vi "SpectrometerSpinCoater_v06.vi"() -> ()   [LabVIEW 2018]
uses:
  <instrlib>/Classes/CCD/Abstract_CCD/Abstract_CCD.lvclass
  TypDef/DeviceQueue_TypeDef.ctl
  TypDef/DeviceQueue_Action.ctl
  TypDef/DataQueue_TypeDef.ctl
  TypDef/DataQueue_Action.ctl
  <vilib>/Utility/error.llb/DialogType.ctl
  <instrlib>/Classes/CCD/Avantes/Avantes.lvclass
  C:/Program Files/National Instruments/LabVIEW 2018/instr.lib/Classes/CCD/Abstract_CCD/Abstract_CCD.lvclass
  <vilib>/Analysis/baseanly.llb/A x Vector.vi
  <vilib>/Instr/_visa.llb/VISA Configure Serial Port (Instr).vi
  <vilib>/Analysis/NI_AALBase.lvlib
panel:
  out "Time.spin":refnum<file>
  out "Meas.spin":refnum<file>
  out "Arduino":bool
  out "NKT":bool
  out "Spectromter":bool
  in  "Abort Button":bool
  in  "Stop Button":bool
  in  "Tab Control":enum32{"Measure", "Settings"}(tab)=enum."Settings"
  in  "Spectra Count":u16
  in  "Measure Spectrum":bool
  out "Action":string
  in  "Preview":bool
  out "XY Graph":T1(graph)
  in  "Frames for Spectrometer":dbl=1.0
  in  "StartSpin_Button":bool
  out "Overall Time":dbl
  in  "Seconds after Spin Stop":dbl[unit]=0.5
  in  "Program Spin Coater\nSpeed (rpm)          Time (s)":dbl[][](array[numeric])
  in  "Record RefSpec":bool
  in  "Record_Darkspec":bool
  in  "Comments":string="Just for testing"
  in  "File Name":string="Temp"
  in  "Save Path":path=path "C:/Users/Timo/Desktop/SpinCoater/Measurement"
  in  "Seconds to Spin Start":dbl[unit]=1.0
  in  "Calculate Frames":bool=TRUE
  in  "Frames":i32
  out "Frame Rate":dbl[unit]
  in  "Integration Time":dbl[unit]=3e-05
  in  "StartMeasurement_Button":bool
  in  "Dividider Get Spectra":u32=1 min=1
  in  "Automatically \nadjust count":bool
  in  "Reset Count\nafter Spin Coating":bool
  in  "Speed":dbl
  in  "Milliseconds":dbl
  in  "Debug":bool
  in  "Port Arduino":refnum<visa-resource-name>="COM6"
  out "Error Arduino":bool caption="Error"
  in  "Init_Arduino":bool=TRUE caption="Init"
  out "Caption_Settings_Arduino":string="Arduino"
  out "Caption_Settings_NKT":string="NKT Laser"
  out "Error_Spectromter":bool caption="Error"
  in  "Init_Spectrometer":bool=TRUE caption="Init"
  out "Caption_Settings_Spectrometer":string="Spectromter"
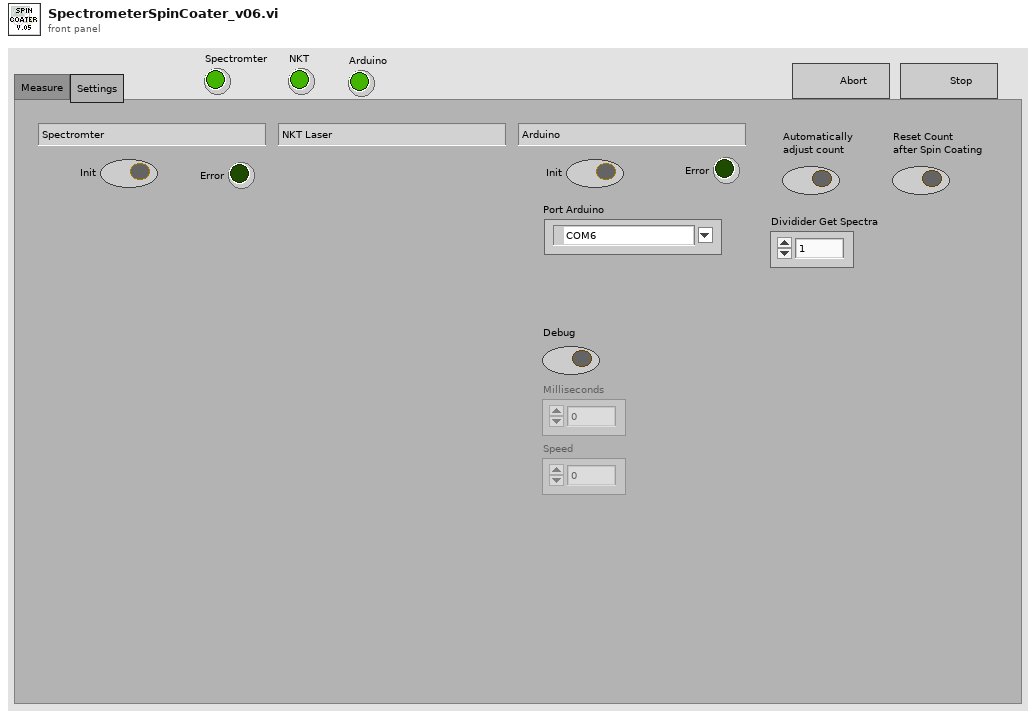
[diagram p1: front panel]
types:
  T1 = cluster{"Wavlength":dbl[unit][], "Image":dbl[]}[]
  T2 = cluster{"Dark":cluster{"Image":dbl[][][], "Frame Size":cluster{"F":i32, "Y":i32, "X":i32}}[], "Ref":cluster{"Image":dbl[][][], "Frame Size":cluster{"F":i32, "Y":i32, "X":i32}}[], "Wavlength":dbl[unit][], "spec":dbl[][]}
  T3 = cluster{"Port Arduino":refnum<visa-resource-name>, "Abstract_CCD.lvclass":refnum<class "Abstract_CCD.lvclass">}
  T4 = typedef "DataQueue_TypeDef.ctl" = cluster{"QueueAction":T5, "Data":cluster{"Image":dbl[][][], "Frame Size":cluster{"F":i32, "Y":i32, "X":i32}}[], "Data_Raw":cluster{"Image":dbl[][][], "Frame Size":cluster{"F":i32, "Y":i32, "X":i32}}[], "Data_Dark":cluster{"Image":dbl[][][], "Frame Size":cluster{"F":i32, "Y":i32, "X":i32}}[], "Data_Ref":cluster{"Image":dbl[][][], "Frame Size":cluster{"F":i32, "Y":i32, "X":i32}}[], "Device Information":string[], "Numeric Control":dbl, "Boolean":bool, "Wavelength":dbl[unit][], "Time":dbl[], "Time Stamp":timestamp, "Numeric Control 2":dbl}
  T5 = typedef "DataQueue_Action.ctl" = enum16{"TimeOut", "Close_Program", "Stop_Measurement", "Measure_InSituSpinCoating", "Measure_Spectrum", "Save_Data", "Set_Ref", "Set_Dark", "Set_Wavelength", "Spectrometer_Measure", "Spectrometer_Preview", "Transfer_Settings"}
  T6 = typedef "DeviceQueue_TypeDef.ctl" = cluster{"QueueAction":T7, "Numeric 1":dbl, "Numeric 2":dbl, "Boolean 1":bool, "Boolean 2":bool, "Spin Program":dbl[][]}
  T7 = typedef "DeviceQueue_Action.ctl" = enum16{"TimeOut", "Close_Program", "Abort", "Spectrometer_Init", "Spectrometer_Close", "Spectrometer_DeviceInformation", "Spectrometer_Measure", "Spectrometer_Preview", "Spectrometer_Abort", "Spectrometer_StartMeasurement", "Spectrometer_GetData", "Spectrometer_StopMeasurement", "Spectrometer_SetIntegrationTime", "Spectrometer_SetFrames", "Spectrometer_SetDarkspec", "Spectrometer_SetReference", "Spectrometer_SetTriggerMode", "Laser_Init", "Laser_Close", "Arduino_Init", "Arduino_Close", "Arduino_LoadProgram", "Arduino_StartProgram", "Arduino_SetSpeed", "Arduino_SetMillis", "Arduino_StopSpin", "Measure_InSitu", "Measure_Spectrum", "Measure_Stop"}
  T8 = enum16{"open", "replace", "create", "open or create", "replace or create", "replace or create with confirmation"}
  T9 = cluster{"Image":dbl[][][], "Frame Size":cluster{"F":i32, "Y":i32, "X":i32}}[]
  T10 = cluster{"Image":dbl[][][], "Frame Size":cluster{"F":i32, "Y":i32, "X":i32}}
  T11 = cluster{"Wavlength":dbl[unit][], "A x Vector":dbl[]}
  T12 = cluster{"Wavlength":dbl[unit][], "A x Vector":dbl[]}[]
  T13 = cluster{u16[][], u16[][], dbl[], "Numeric Control":dbl, "Numeric Control 2":dbl}
  T14 = typedef "DialogType.ctl" = u16
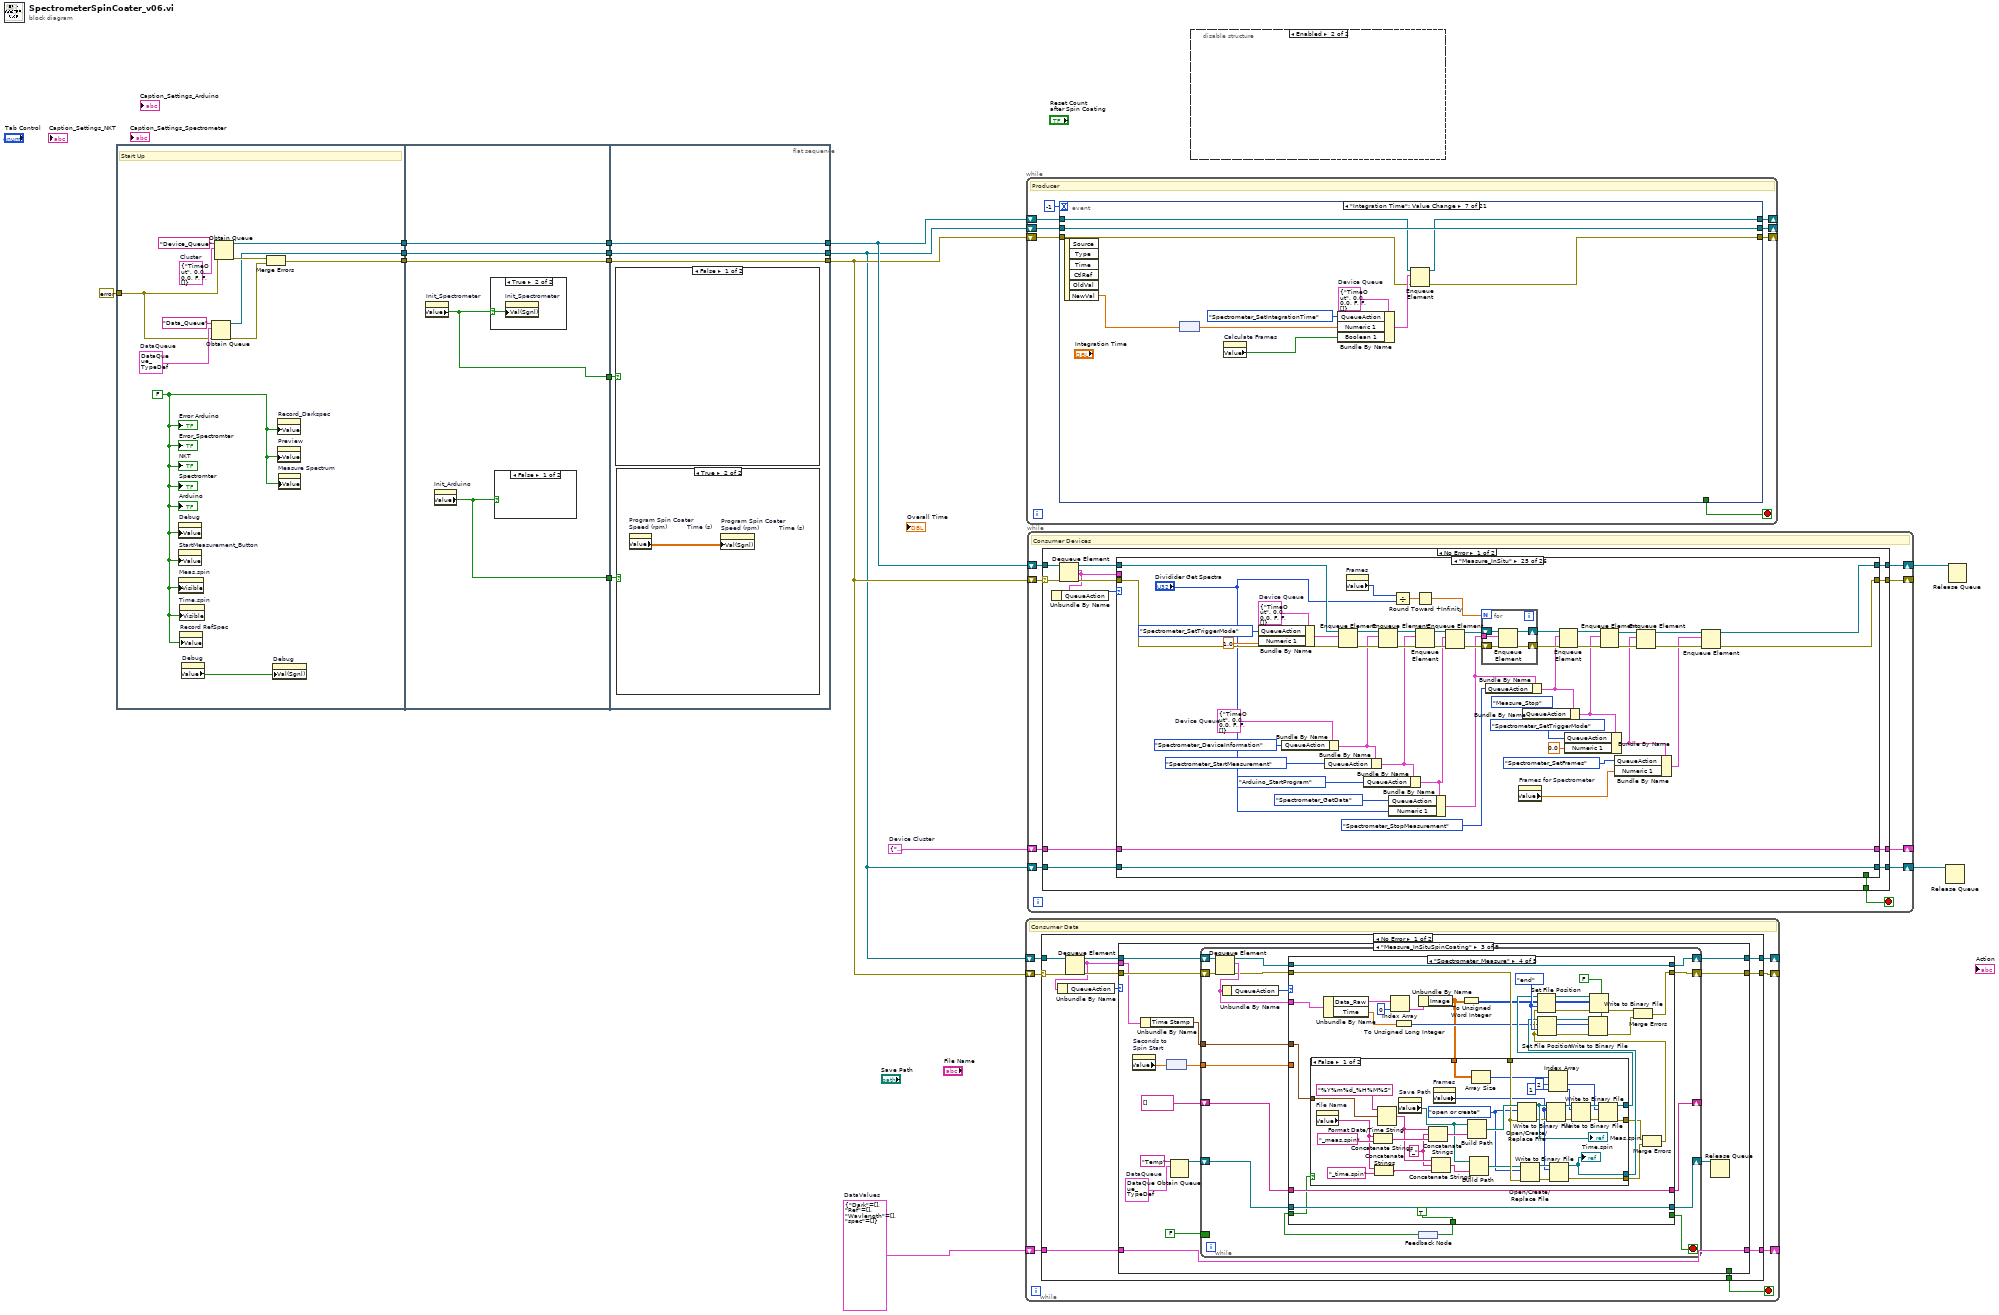
[diagram p0: block diagram]
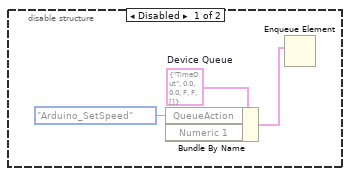
[diagram p2: hidden frame]
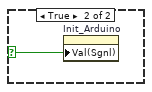
[diagram p3: hidden frame]
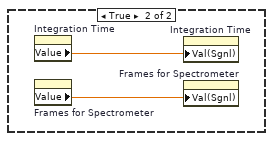
[diagram p6: hidden frame]
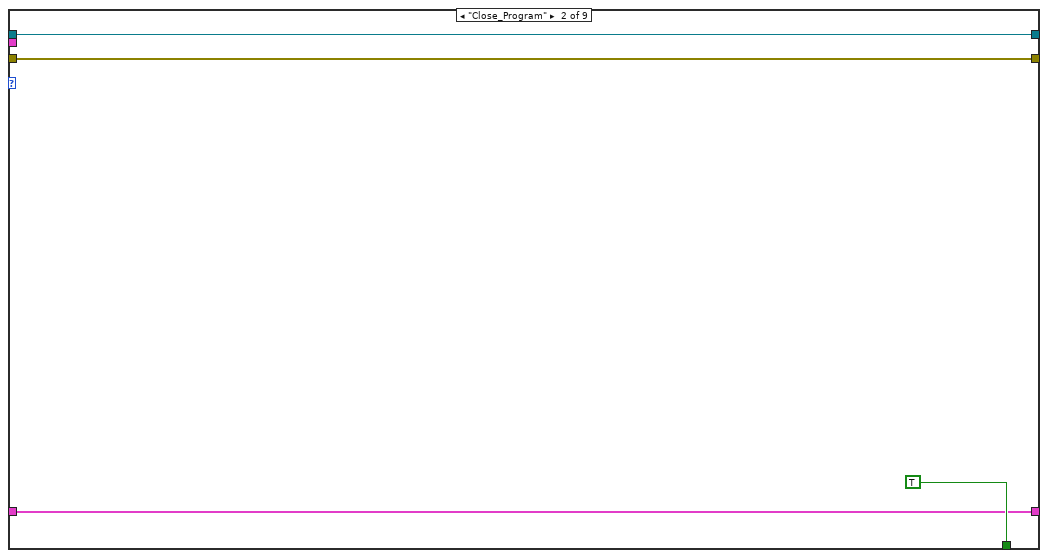
[diagram p8: hidden frame]
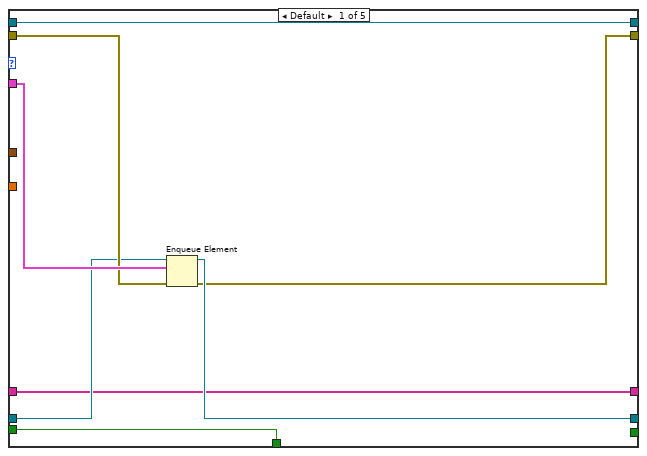
[diagram p9: hidden frame]
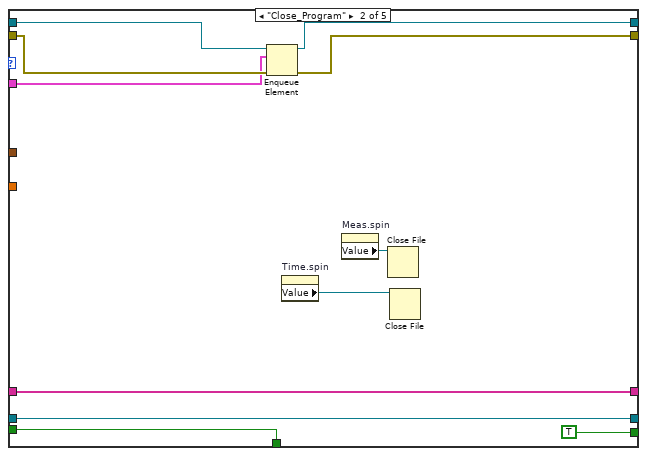
[diagram p10: hidden frame]
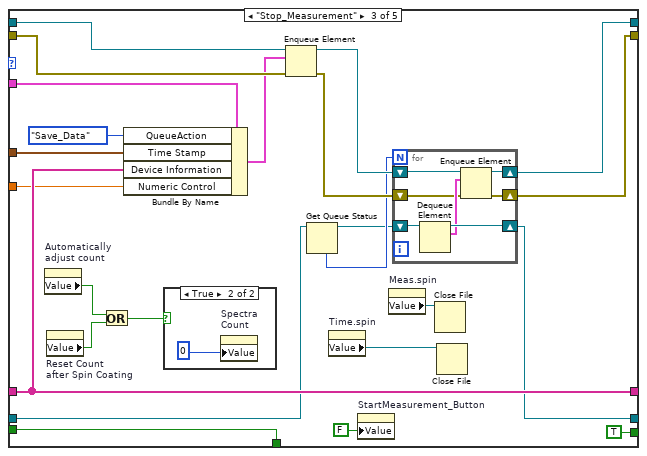
[diagram p11: hidden frame]
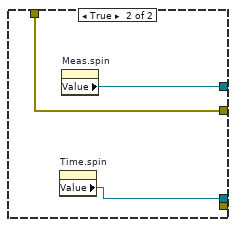
[diagram p13: hidden frame]
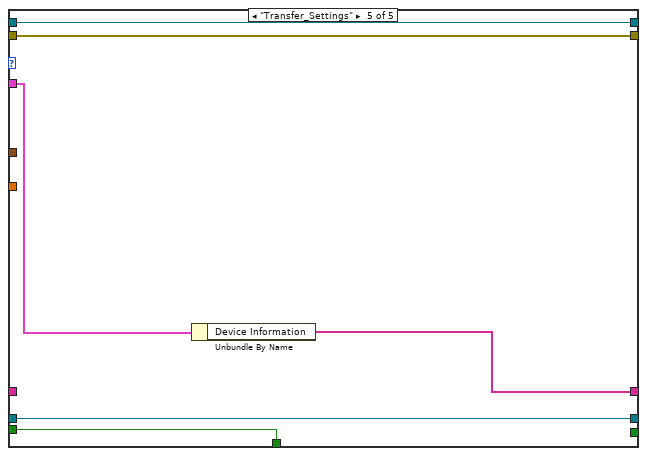
[diagram p14: hidden frame]
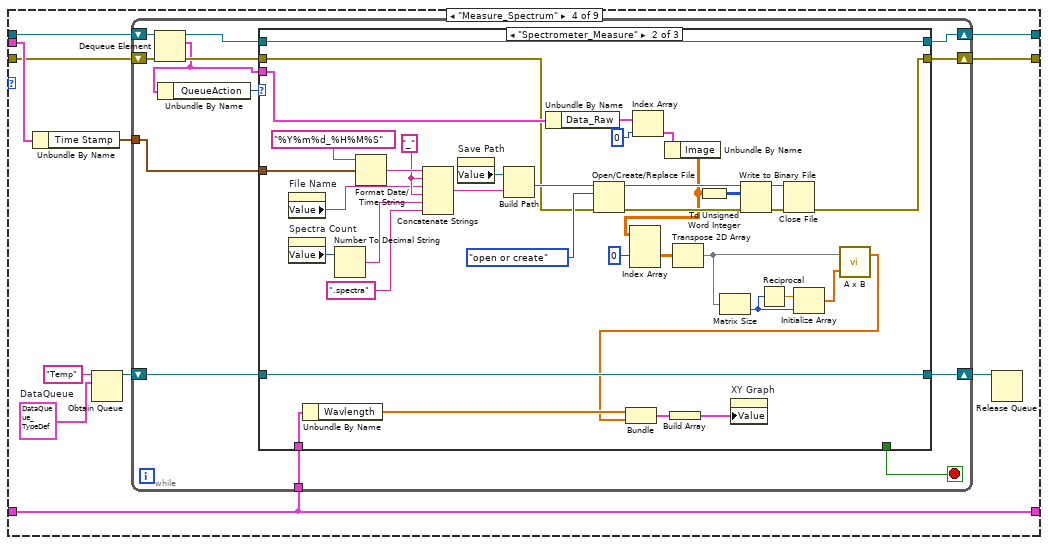
[diagram p15: hidden frame]
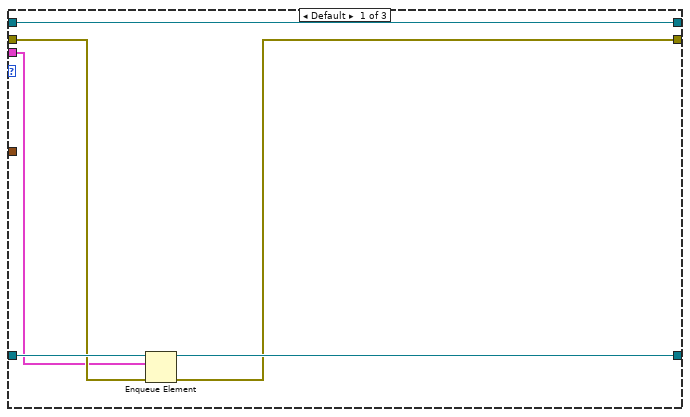
[diagram p16: hidden frame]
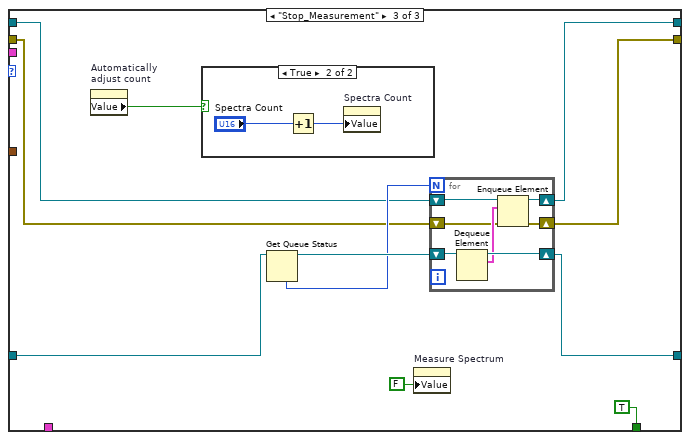
[diagram p17: hidden frame]
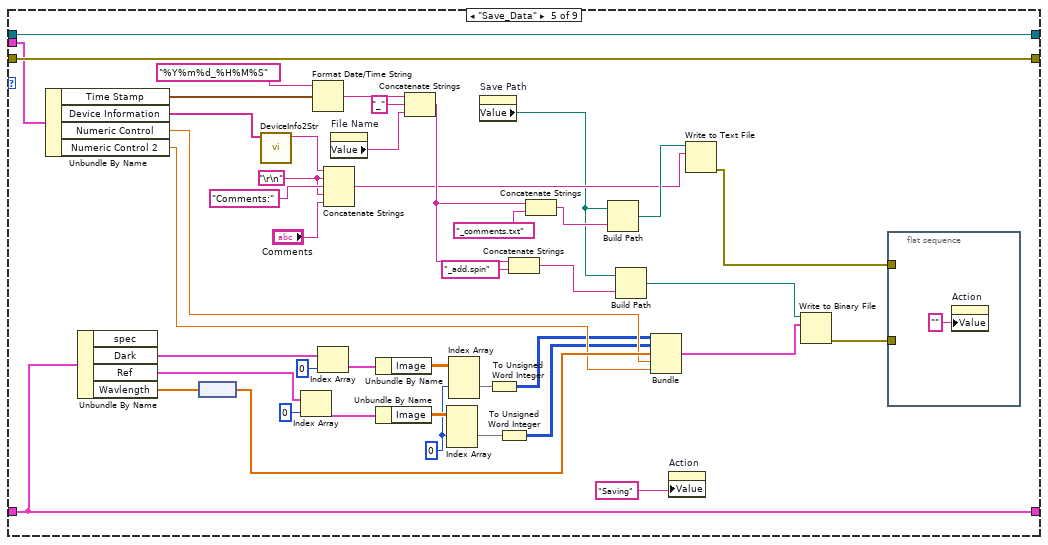
[diagram p19: hidden frame]
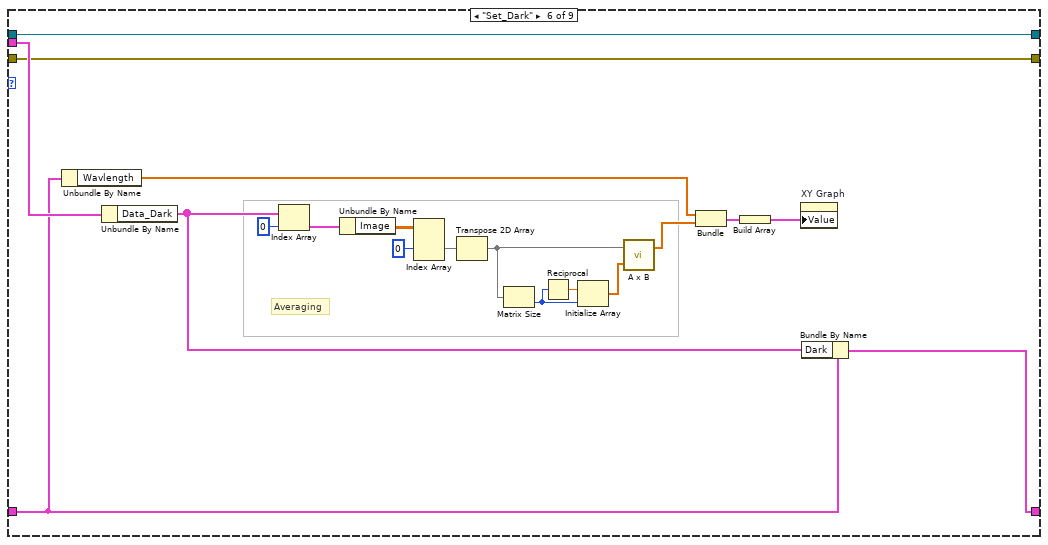
[diagram p20: hidden frame]
diagram:
  w6 = T2 {"Dark"=[], "Ref"=[], "Wavlength"=[], "spec"=[]}  # DataValues
  w11 = T3 {"Port Arduino"="", "Abstract_CCD.lvclass"=refnum}  # Device Cluster
  n1 = flat-sequence {
    tunnel: errorcluster {"status"=FALSE, "code"=0, "source"=""} ("error constant") -> [w23]
    tunnel: [w26] -> w15
    tunnel: [w20] -> w14
    tunnel: [w19] -> w13
    tunnel: w15 -> [w33]
    tunnel: w14 -> [w32]
    tunnel: w13 -> [w31]
    tunnel: [w33] -> w5
    tunnel: [w32] -> w4
    tunnel: [w31] -> w3
    tunnel: [w30] -> w2
    tunnel: [w29] -> w1
    tunnel: [w38] -> w8
    tunnel: [w39] -> w7
    tunnel: [w40] -> w12
    tunnel: w5 -> [w40]
    tunnel: w4 -> [w39]
    tunnel: w3 -> [w38]
    tunnel: w2 -> [w37]
    tunnel: w1 -> [w36]
    frame #0 {
      w24 = T4 {"QueueAction"=enum."TimeOut", "Data"=[], "Data_Raw"=[], "Data_Dark"=[], "Data_Ref"=[], "Device Information"=[], "Numeric Control"=0.0, "Boolean"=FALSE, "Wavelength"=[], "Time"=[], "Time Stamp"=timestamp(0 s since 1904-01-01), "Numeric Control 2"=0.0}  # DataQueue
      w27 = T6 {"QueueAction"=enum."TimeOut", "Numeric 1"=0.0, "Numeric 2"=0.0, "Boolean 1"=FALSE, "Boolean 2"=FALSE, "Spin Program"=[]}  # Cluster
      w18 = FALSE ("Error Arduino")
      # "Start Up"
      n2 = property on="Debug" class="Bool (strict)"("Value"=w18) -> ()  [unwired: 2 in, 2 out]
      n3 = property on="StartMeasurement_Button" class="Bool (strict)"("Value"=w18) -> ()  [unwired: 2 in, 2 out]
      n4 = property on="Meas.spin" class="Ref (strict)"("Visible"=w18) -> ()  [unwired: 2 in, 2 out]
      n5 = property on="Time.spin" class="Ref (strict)"("Visible"=w18) -> ()  [unwired: 2 in, 2 out]
      n6 = property on="Record RefSpec" class="Bool (strict)"("Value"=w18) -> ()  [unwired: 2 in, 2 out]
      n7 = property on="Debug" class="Bool (strict)"() -> ("Value"=w17:bool)  [unwired: 2 in, 2 out]
      n8 = Obtain Queue(name (unnamed)="Data_Queue", element data type=w24, error in (no error)=w23) -> (queue out=w20:refnum<queue>, error out=w21:errorcluster)  [unwired: 2 in, 1 out]
      n9 = Obtain Queue(name (unnamed)="Device_Queue", element data type=w27, error in (no error)=w23) -> (queue out=w26:refnum<queue>, error out=w22:errorcluster)  [unwired: 2 in, 1 out]
      n10 = Merge Errors(w22, w21) -> (w19:errorcluster)
      n11 = property on="Debug" class="Bool (strict)"("Val(Sgnl)"=w17) -> ()  [unwired: 2 in, 2 out]
      n12 = property on="Record_Darkspec" class="Bool (strict)"("Value"=w18) -> ()  [unwired: 2 in, 2 out]
      n13 = property on="Preview" class="Bool (strict)"("Value"=w18) -> ()  [unwired: 2 in, 2 out]
      n14 = property on="Measure Spectrum" class="Bool (strict)"("Value"=w18) -> ()  [unwired: 2 in, 2 out]
      "Error_Spectromter" <- w18
      "Error Arduino" <- w18
      "Spectromter" <- w18
      "NKT" <- w18
      "Arduino" <- w18
    }
    frame #1 {
      n15 = property on="Init_Spectrometer" class="Bool (strict)"() -> ("Value"=w30:bool)  [unwired: 2 in, 2 out]
      n16 = property on="Init_Arduino" class="Bool (strict)"() -> ("Value"=w29:bool)  [unwired: 2 in, 2 out]
      n17 = case shown="True" w30 {
        selector: w30 -> [_ w35]
        frame False {
        }
        frame True {
          n18 = property on="Init_Spectrometer" class="Bool (strict)"("Val(Sgnl)"=w35) -> ()  [unwired: 2 in, 2 out]
        }
      }
      n19 = case shown="False" w29 {
        selector: w29 -> [_ w34]
        frame False {
        }
        frame True {
          n20 = property on="Init_Arduino" class="Bool (strict)"("Val(Sgnl)"=w34) -> ()  [unwired: 2 in, 2 out]
        }
      }
    }
    frame #2 {
      n21 = case shown="False" w37 {
        frame False {
        }
        frame True {
          n22 = property on="Integration Time" class="DigNum (strict)"() -> ("Value"=w42:dbl[unit])  [unwired: 2 in, 2 out]
          n23 = property on="Frames for Spectrometer" class="DigNum (strict)"() -> ("Value"=w43:dbl)  [unwired: 2 in, 2 out]
          n24 = property on="Integration Time" class="DigNum (strict)"("Val(Sgnl)"=w42) -> ()  [unwired: 2 in, 2 out]
          n25 = property on="Frames for Spectrometer" class="DigNum (strict)"("Val(Sgnl)"=w43) -> ()  [unwired: 2 in, 2 out]
        }
      }
      n26 = case shown="True" w36 {
        frame False {
        }
        frame True {
          n27 = property on="Program Spin Coater\nSpeed (rpm)          Time (s)" class="Arr (strict)"() -> ("Value"=w41:dbl[][])  [unwired: 2 in, 2 out]
          n28 = property on="Program Spin Coater\nSpeed (rpm)          Time (s)" class="Arr (strict)"("Val(Sgnl)"=w41) -> ()  [unwired: 2 in, 2 out]
        }
      }
    }
  }
  n29 = while {
    shift-right: [w44] -> _
    shift-left: w8 -> [w50]
    shift-right: [w45] -> _
    shift-left: w7 -> [w49]
    shift-right: [w46] -> _
    shift-left: w6 -> [w48]
    stop <- w47 stop-if-true
    # "Consumer Data"
    n30 = case shown="No Error" w50 {
      selector: w50 -> [w61 w416]
      tunnel: w49 -> [w60 w417]
      tunnel: w48 -> [w58 w414]
      tunnel: [w57 _] -> w47
      tunnel: [w56 w414] -> w46
      tunnel: [w55 w417] -> w45
      tunnel: [w53 w415] -> w44
      frame No Error {
        n31 = Dequeue Element(queue=w60, error in (no error)=w61) -> (queue out=w54:refnum<queue>, element=w51:T4, error out=w52:errorcluster)  [unwired: 1 in, 1 out]
        n32 = Unbundle By Name(w51) -> ("QueueAction"=w59:T5)
        n33 = case shown="\"Measure_InSituSpinCoating\"" w59 {
          tunnel: w58 -> [w62 w67 w73 w225 w325 w368 w377 w399 w410]
          tunnel: [_ TRUE _ _ _ _ _ _ _] -> w57
          tunnel: [w62 w67 w73 w225 w325 w372 w391 w398 w410] -> w56
          tunnel: [w64 w66 w83 w231 w355 w373 w392 w395 w413] -> w55
          tunnel: w54 -> [w64 w66 w81 w233 w355 w373 w392 w395 w413]
          tunnel: [w63 w65 w82 w230 w354 w374 w393 w396 w412] -> w53
          tunnel: w52 -> [w63 w65 w80 w234 w354 w374 w393 w396 w412]
          tunnel: w51 -> [_ _ w75 w235 w341 w375 w394 w397 w411]
          frame "TimeOut", Default {
          }
          frame "Close_Program" {
          }
          frame "Measure_InSituSpinCoating" {
            w78 = T4 {"QueueAction"=enum."TimeOut", "Data"=[], "Data_Raw"=[], "Data_Dark"=[], "Data_Ref"=[], "Device Information"=[], "Numeric Control"=0.0, "Boolean"=FALSE, "Wavelength"=[], "Time"=[], "Time Stamp"=timestamp(0 s since 1904-01-01), "Numeric Control 2"=0.0}  # DataQueue
            n34 = property on="Seconds to\nSpin Start" class="DigNum (strict)"() -> ("Value"=w70:dbl[unit])  [unwired: 2 in, 2 out]
            n35 = Unbundle By Name(w75) -> ("Time Stamp"=w74:timestamp)
            n36 = node(w70) -> (w69:dbl)
            n37 = Obtain Queue(name (unnamed)="Temp", element data type=w78) -> (queue out=w77:refnum<queue>)  [unwired: 3 in, 2 out]
            n38 = while {
              shift-right: [w91] -> w83
              shift-left: w81 -> [w100]
              shift-right: [w92] -> w82
              shift-left: w80 -> [w99]
              shift-right: [w93] -> w76
              shift-left: w77 -> [w94]
              tunnel: w74 -> [w87]
              shift-right: [w88] -> _
              shift-left: string[] [] ("Device Information") -> [w89]
              border: FALSE -> [_]
              tunnel: w69 -> [w84]
              stop <- w90 stop-if-true
              n39 = Dequeue Element(queue=w100, error in (no error)=w99) -> (queue out=w95:refnum<queue>, element=w97:T4, error out=w96:errorcluster)  [unwired: 1 in, 1 out]
              n40 = Unbundle By Name(w97) -> ("QueueAction"=w98:T5)
              n41 = feedback #1() -> (w86:bool)
              n42 = case shown="\"Spectrometer_Measure\"" w98 {
                tunnel: w97 -> [w108 w117 w142 w179 w223]
                tunnel: w96 -> [w107 w118 w139 w170 w220]
                tunnel: w95 -> [w103 w119 w138 w178 w221]
                tunnel: w94 -> [w106 w114 w133 w167 w224]
                tunnel: [w105 w114 w130 w167 w224] -> w93
                tunnel: [w104 w115 w129 w168 w220] -> w92
                tunnel: [w103 w116 w128 w178 w221] -> w91
                tunnel: [_ TRUE TRUE _ _] -> w90
                tunnel: w89 -> [w102 w112 w140 w165 _]
                tunnel: [w102 w112 w140 w165 w222] -> w88
                tunnel: w87 -> [_ _ w141 w180 _]
                tunnel: w86 -> [w101 w111 w127 w163 w219]
                tunnel: [w101 w111 w127 TRUE w219] -> w85
                tunnel: w84 -> [_ _ w124 _ _]
                frame Default {
                  n43 = Enqueue Element(queue=w106, element=w108, error in (no error)=w107) -> (queue out=w105:refnum<queue>, error out=w104:errorcluster)  [unwired: 1 in, 1 out]
                }
                frame "Close_Program" {
                  n44 = Enqueue Element(queue=w119, element=w117, error in (no error)=w118) -> (queue out=w116:refnum<queue>, error out=w115:errorcluster)  [unwired: 1 in, 1 out]
                  n45 = property on="Time.spin" class="Ref (strict)"() -> ("Value"=w109:refnum<file>)  [unwired: 2 in, 2 out]
                  n46 = property on="Meas.spin" class="Ref (strict)"() -> ("Value"=w110:refnum<file>)  [unwired: 2 in, 2 out]
                  n47 = Close File(refnum=w110) -> ()  [unwired: 1 in, 2 out]
                  n48 = Close File(refnum=w109) -> ()  [unwired: 1 in, 2 out]
                }
                frame "Stop_Measurement" {
                  n49 = property on="Automatically \nadjust count" class="Bool (strict)"() -> ("Value"=w121:bool)  [unwired: 2 in, 2 out]
                  n50 = property on="Reset Count\nafter Spin Coating" class="Bool (strict)"() -> ("Value"=w122:bool)  [unwired: 2 in, 2 out]
                  n51 = Or(x=w121, y=w122) -> (x .or. y?=w120:bool)
                  n52 = Bundle By Name(cluster=w142, "QueueAction"=DataQueue_Action."Save_Data", "Time Stamp"=w141, "Device Information"=w140, "Numeric Control"=w124) -> (w137:T4)
                  n53 = case shown="True" w120 {
                    frame False {
                    }
                    frame True {
                      n54 = property on="Spectra \nCount" class="DigNum (strict)"("Value"=u16 0 ("Spectra Count")) -> ()  [unwired: 2 in, 2 out]
                    }
                  }
                  n55 = Enqueue Element(queue=w138, element=w137, error in (no error)=w139) -> (queue out=w135:refnum<queue>, error out=w134:errorcluster)  [unwired: 1 in, 1 out]
                  n56 = Get Queue Status(queue=w133) -> (queue out=w131:refnum<queue>, # elements in queue=w132:i32)  [unwired: 2 in, 6 out]
                  n57 = property on="Time.spin" class="Ref (strict)"() -> ("Value"=w125:refnum<file>)  [unwired: 2 in, 2 out]
                  n58 = property on="StartMeasurement_Button" class="Bool (strict)"("Value"=FALSE ("StartMeasurement_Button")) -> ()  [unwired: 2 in, 2 out]
                  n59 = property on="Meas.spin" class="Ref (strict)"() -> ("Value"=w126:refnum<file>)  [unwired: 2 in, 2 out]
                  n60 = for {
                    N: w132 -> [_]
                    shift-right: [w150] -> w130
                    shift-left: w131 -> [w151]
                    shift-right: [w147] -> w128
                    shift-left: w135 -> [w148]
                    shift-right: [w145] -> w129
                    shift-left: w134 -> [w146]
                    n61 = Dequeue Element(queue=w151) -> (queue out=w150:refnum<queue>, element=w149:T4)  [unwired: 2 in, 2 out]
                    n62 = Enqueue Element(queue=w148, element=w149, error in (no error)=w146) -> (queue out=w147:refnum<queue>, error out=w145:errorcluster)  [unwired: 1 in, 1 out]
                  }
                  n63 = Close File(refnum=w126) -> ()  [unwired: 1 in, 2 out]
                  n64 = Close File(refnum=w125) -> ()  [unwired: 1 in, 2 out]
                }
                frame "Spectrometer_Measure" {
                  w153 = FALSE ("prepend array or string size? (T)")
                  w166 = enum16{"start", "end", "current"}."end" ("from (0:start)")
                  n65 = Unbundle By Name(w179) -> ("Data_Raw"=w175:T9, "Time"=w169:dbl[])
                  n66 = Index Array(array=w175, index=0) -> (element=w174:T10)
                  n67 = To Unsigned Long Integer(number=w169) -> (unsigned 32bit integer=w155:u32[])
                  n68 = Unbundle By Name(w174) -> ("Image"=w152:dbl[][][])
                  n69 = case shown="False" w163 {
                    tunnel: w180 -> [w212 _]
                    tunnel: w170 -> [w207 w218]
                    tunnel: [w193 w218] -> w157
                    tunnel: [w181 _] -> w158
                    tunnel: [w192 w217] -> w160
                    tunnel: [w182 w216] -> w159
                    tunnel: w152 -> [w190 _]
                    frame False {
                      w202 = T8."open or create" ("operation (0:open)")
                      w201 = "_" ("string")
                      n70 = property on="File Name" class="Str"() -> ("Value"=w210:string)  [unwired: 2 in, 2 out]
                      n71 = Concatenate Strings(w210, "_meas.spin" ("string")) -> (w213:string)
                      n72 = Concatenate Strings(w210, "_time.spin" ("string")) -> (w205:string)
                      n73 = Format Date/Time String(time format string (%c)="%Y%m%d_%H%M%S", seconds (now)=w212) -> (date/time string=w206:string)  [unwired: 1 in]
                      n74 = property on="Save Path" class="Path"() -> ("Value"=w184:path)  [unwired: 2 in, 2 out]
                      n75 = Concatenate Strings(w206, w201, w213) -> (w211:string)
                      n76 = Concatenate Strings(w206, w201, w205) -> (w204:string)
                      n77 = property on="Frames" class="DigNum (strict)"() -> ("Value"=w183:i32)  [unwired: 2 in, 2 out]
                      n78 = Build Path(base path=w184, name or relative path=w211) -> (appended path=w208:path)
                      n79 = Build Path(base path=w184, name or relative path=w204) -> (appended path=w203:path)
                      n80 = Array Size(array=w190) -> (size(s)=w189:i32[])
                      n81 = Open/Create/Replace File(file path (use dialog)=w208, error in=w207, operation (0:open)=w202) -> (refnum out=w200:refnum<file>, error out=w199:errorcluster)  [unwired: 3 in, 1 out]
                      "Meas.spin" <- w200
                      n82 = Open/Create/Replace File(file path (use dialog)=w203, error in=w207, operation (0:open)=w202) -> (refnum out=w198:refnum<file>, error out=w197:errorcluster)  [unwired: 3 in, 1 out]
                      n83 = Write to Binary File(file (use dialog)=w200, data=w183, error in=w199) -> (refnum out=w196:refnum<file>, error out=w195:errorcluster)  [unwired: 3 in, 1 out]
                      n84 = Index Array(array=w189, index #1=2 ("index"), index #2=1 ("index")) -> (element #1=w185:i32, element #2=w186:i32)
                      n85 = Write to Binary File(file (use dialog)=w198, data=w183, error in=w197) -> (refnum out=w182:refnum<file>, error out=w181:errorcluster)  [unwired: 3 in, 1 out]
                      "Time.spin" <- w182
                      n86 = Write to Binary File(file (use dialog)=w196, data=w186, error in=w195) -> (refnum out=w191:refnum<file>, error out=w194:errorcluster)  [unwired: 3 in, 1 out]
                      n87 = Write to Binary File(file (use dialog)=w191, data=w185, error in=w194) -> (refnum out=w192:refnum<file>, error out=w193:errorcluster)  [unwired: 3 in, 1 out]
                    }
                    frame True {
                      n88 = property on="Time.spin" class="Ref (strict)"() -> ("Value"=w216:refnum<file>)  [unwired: 2 in, 2 out]
                      n89 = property on="Meas.spin" class="Ref (strict)"() -> ("Value"=w217:refnum<file>)  [unwired: 2 in, 2 out]
                    }
                  }
                  n90 = To Unsigned Word Integer(number=w152) -> (unsigned 16bit integer=w154:u16[][][])
                  n91 = Merge Errors(w157, w158) -> (w156:errorcluster)
                  n92 = Set File Position(refnum=w160, from (0:start)=w166, error in=w156) -> (refnum out=w172:refnum<file>, error out=w171:errorcluster)  [unwired: 1 in]
                  n93 = Set File Position(refnum=w159, from (0:start)=w166, error in=w156) -> (refnum out=w177:refnum<file>, error out=w176:errorcluster)  [unwired: 1 in]
                  n94 = Write to Binary File(file (use dialog)=w177, data=w155, error in=w176, 5:w153) -> (error out=w161:errorcluster)  [unwired: 2 in, 2 out]
                  n95 = Write to Binary File(file (use dialog)=w172, data=w154, error in=w171, 5:w153) -> (error out=w162:errorcluster)  [unwired: 2 in, 2 out]
                  n96 = Merge Errors(w162, w161) -> (w168:errorcluster)
                }
                frame "Transfer_Settings" {
                  n97 = Unbundle By Name(w223) -> ("Device Information"=w222:string[])
                }
              }
              n98 = feedback-in #1(w85) -> ()
            }
            n99 = Release Queue(queue=w76) -> ()  [unwired: 2 in, 3 out]
          }
          frame "Measure_Spectrum" {
            w228 = T4 {"QueueAction"=enum."TimeOut", "Data"=[], "Data_Raw"=[], "Data_Dark"=[], "Data_Ref"=[], "Device Information"=[], "Numeric Control"=0.0, "Boolean"=FALSE, "Wavelength"=[], "Time"=[], "Time Stamp"=timestamp(0 s since 1904-01-01), "Numeric Control 2"=0.0}  # DataQueue
            n100 = Unbundle By Name(w235) -> ("Time Stamp"=w232:timestamp)
            n101 = Obtain Queue(name (unnamed)="Temp", element data type=w228) -> (queue out=w227:refnum<queue>)  [unwired: 3 in, 2 out]
            n102 = while {
              shift-right: [w239] -> w231
              shift-left: w233 -> [w247]
              shift-right: [w240] -> w230
              shift-left: w234 -> [w248]
              tunnel: w232 -> [w237]
              shift-right: [w241] -> w226
              shift-left: w227 -> [w243]
              tunnel: w225 -> [w236]
              stop <- w238 stop-if-true
              n103 = Dequeue Element(queue=w247, error in (no error)=w248) -> (queue out=w245:refnum<queue>, element=w242:T4, error out=w244:errorcluster)  [unwired: 1 in, 1 out]
              n104 = Unbundle By Name(w242) -> ("QueueAction"=w246:T5)
              n105 = case shown="\"Spectrometer_Measure\"" w246 {
                tunnel: w245 -> [w249 w267 w298]
                tunnel: w244 -> [w252 w277 w297]
                tunnel: w243 -> [w254 w289 w300]
                tunnel: w242 -> [w250 w291 _]
                tunnel: [w253 w289 w296] -> w241
                tunnel: [w251 w268 w294] -> w240
                tunnel: [w249 w267 w295] -> w239
                tunnel: [_ _ TRUE] -> w238
                tunnel: w237 -> [_ w288 _]
                tunnel: w236 -> [_ w259 _]
                frame Default {
                  n106 = Enqueue Element(queue=w254, element=w250, error in (no error)=w252) -> (queue out=w253:refnum<queue>, error out=w251:errorcluster)  [unwired: 1 in, 1 out]
                }
                frame "Spectrometer_Measure" {
                  w285 = "_"
                  n107 = property on="File Name" class="Str"() -> ("Value"=w284:string)  [unwired: 2 in, 2 out]
                  n108 = property on="Spectra Count" class="DigNum (strict)"() -> ("Value"=w290:u16)  [unwired: 2 in, 2 out]
                  n109 = Unbundle By Name(w259) -> ("Wavlength"=w256:dbl[unit][])
                  n110 = Number To Decimal String(number=w290) -> (decimal integer string=w283:string)  [unwired: 1 in]
                  n111 = Format Date/Time String(time format string (%c)="%Y%m%d_%H%M%S", seconds (now)=w288) -> (date/time string=w286:string)  [unwired: 1 in]
                  n112 = Concatenate Strings(w286, w285, w284, w285, w283, ".spectra" ("string")) -> (w281:string)
                  n113 = property on="Save Path" class="Path"() -> ("Value"=w280:path)  [unwired: 2 in, 2 out]
                  n114 = Build Path(base path=w280, name or relative path=w281) -> (appended path=w279:path)
                  n115 = Unbundle By Name(w291) -> ("Data_Raw"=w274:T9)
                  n116 = Open/Create/Replace File(file path (use dialog)=w279, error in=w277, operation (0:open)=T8."open or create") -> (refnum out=w276:refnum<file>, error out=w275:errorcluster)  [unwired: 3 in, 1 out]
                  n117 = Index Array(array=w274, index=0) -> (element=w272:T10)
                  n118 = Unbundle By Name(w272) -> ("Image"=w260:dbl[][][])
                  n119 = Index Array(array=w260, index (dim 1)=0 ("disabled index (row)")) -> (element=w266:dbl[][])  [unwired: 2 in]
                  n120 = Transpose 2D Array(2D array=w266) -> (transposed array=w263:dbl[][])
                  n121 = To Unsigned Word Integer(number=w260) -> (unsigned 16bit integer=w271:u16[][][])
                  n122 = Matrix Size(0:w263) -> (2:w264:i32)  [unwired: 1 out]
                  n123 = Write to Binary File(file (use dialog)=w276, data=w271, error in=w275) -> (refnum out=w269:refnum<file>, error out=w270:errorcluster)  [unwired: 3 in, 1 out]
                  n124 = Reciprocal(x=w264) -> (1/x=w265:dbl)
                  n125 = Close File(refnum=w269, error in=w270) -> (error out=w268:errorcluster)  [unwired: 1 out]
                  n126 = Initialize Array(w265, w264) -> (w262:dbl[])
                  n127 = call-poly <vilib>:"A x B.vi"("Vector"=w262, "A"=w263) -> ("A x Vector"=w255:dbl[])  [unwired: 1 out]
                  n128 = Bundle("Wavlength"=w256, "A x Vector"=w255) -> (w258:T11)  [unwired: 1 in]
                  n129 = Build Array(w258) -> (w257:T12)
                  n130 = property on="XY Graph" class="XYGraph (strict)"("Value"=w257) -> ()  [unwired: 2 in, 2 out]
                }
                frame "Stop_Measurement" {
                  n131 = property on="Automatically \nadjust count" class="Bool (strict)"() -> ("Value"=w292:bool)  [unwired: 2 in, 2 out]
                  n132 = case shown="True" w292 {
                    frame False {
                    }
                    frame True {
                      n133 = Increment(x="Spectra Count") -> (x+1=w303:u16)
                      n134 = property on="Spectra Count" class="DigNum (strict)"("Value"=w303) -> ()  [unwired: 2 in, 2 out]
                    }
                  }
                  n135 = Get Queue Status(queue=w300) -> (queue out=w301:refnum<queue>, # elements in queue=w299:i32)  [unwired: 2 in, 6 out]
                  n136 = property on="Measure Spectrum" class="Bool (strict)"("Value"=FALSE ("Measure Spectrum")) -> ()  [unwired: 2 in, 2 out]
                  n137 = for {
                    N: w299 -> [_]
                    shift-right: [w310] -> w296
                    shift-left: w301 -> [w311]
                    shift-right: [w307] -> w295
                    shift-left: w298 -> [w308]
                    shift-right: [w305] -> w294
                    shift-left: w297 -> [w306]
                    n138 = Dequeue Element(queue=w311) -> (queue out=w310:refnum<queue>, element=w309:T4)  [unwired: 2 in, 2 out]
                    n139 = Enqueue Element(queue=w308, element=w309, error in (no error)=w306) -> (queue out=w307:refnum<queue>, error out=w305:errorcluster)  [unwired: 1 in, 1 out]
                  }
                }
              }
            }
            n140 = Release Queue(queue=w226) -> ()  [unwired: 2 in, 3 out]
          }
          frame "Save_Data" {
            w327 = "\r\n"
            w314 = 0 ("index (page)")
            n141 = Unbundle By Name(w341) -> ("Time Stamp"=w339:timestamp, "Device Information"=w330:string[], "Numeric Control"=w324:dbl, "Numeric Control 2"=w323:dbl)
            n142 = Unbundle By Name(w325) -> ("Dark"=w351:T9, "Ref"=w349:T9, "Wavlength"=w353:dbl[unit][])  [unwired: 1 out]
            n143 = node(w353) -> (w342:dbl[])
            n144 = call "DeviceInfo2Str.vi"("Device Information"=w330) -> ("String"=w329:string)  [unwired: 10 in]
            n145 = Index Array(array=w349, index=0) -> (element=w347:T10)
            n146 = Format Date/Time String(time format string (%c)="%Y%m%d_%H%M%S", seconds (now)=w339) -> (date/time string=w338:string)  [unwired: 1 in]
            n147 = Index Array(array=w351, index=0) -> (element=w348:T10)
            n148 = Concatenate Strings(w329, w327, "Comments:" ("string"), w327, "Comments") -> (w322:string)
            n149 = property on="File Name" class="Str"() -> ("Value"=w320:string)  [unwired: 2 in, 2 out]
            n150 = Unbundle By Name(w348) -> ("Image"=w346:dbl[][][])
            n151 = Unbundle By Name(w347) -> ("Image"=w345:dbl[][][])
            n152 = Concatenate Strings(w338, "_" ("string"), w320) -> (w336:string)
            n153 = Index Array(array=w345, index (dim 1)=w314) -> (element=w343:dbl[][])  [unwired: 2 in]
            n154 = Index Array(array=w346, index (dim 1)=w314) -> (element=w344:dbl[][])  [unwired: 2 in]
            n155 = property on="Save Path" class="Path"() -> ("Value"=w319:path)  [unwired: 2 in, 2 out]
            n156 = To Unsigned Word Integer(number=w344) -> (unsigned 16bit integer=w313:u16[][])
            n157 = To Unsigned Word Integer(number=w343) -> (unsigned 16bit integer=w312:u16[][])
            n158 = Concatenate Strings(w336, "_add.spin" ("string")) -> (w334:string)
            n159 = Concatenate Strings(w336, "_comments.txt" ("string")) -> (w333:string)
            n160 = Build Path(base path=w319, name or relative path=w333) -> (appended path=w332:path)
            n161 = Build Path(base path=w319, name or relative path=w334) -> (appended path=w318:path)
            n162 = Bundle(w313, w312, w342, "Numeric Control"=w324, "Numeric Control 2"=w323) -> (w317:T13)  [unwired: 1 in]
            n163 = property on="Action" class="Str"("Value"="Saving" ("Action")) -> ()  [unwired: 2 in, 2 out]
            n164 = Write to Text File(file (use dialog)=w332, text=w322) -> (error out=w316:errorcluster)  [unwired: 2 in, 2 out]
            n165 = Write to Binary File(file (use dialog)=w318, data=w317) -> (error out=w315:errorcluster)  [unwired: 4 in, 2 out]
            n166 = flat-sequence {
              tunnel: w316 -> [_]
              tunnel: w315 -> [_]
              frame #0 {
                n167 = property on="Action" class="Str"("Value"="" ("Action")) -> ()  [unwired: 2 in, 2 out]
              }
            }
          }
          frame "Set_Dark" {
            # "Averaging"
            n168 = Unbundle By Name(w368) -> ("Wavlength"=w367:dbl[unit][])
            n169 = Unbundle By Name(w375) -> ("Data_Dark"=w365:T9)
            n170 = Index Array(array=w365, index=0) -> (element=w370:T10)
            n171 = Unbundle By Name(w370) -> ("Image"=w364:dbl[][][])
            n172 = Index Array(array=w364, index (dim 1)=0 ("disabled index (row)")) -> (element=w362:dbl[][])  [unwired: 2 in]
            n173 = Transpose 2D Array(2D array=w362) -> (transposed array=w359:dbl[][])
            n174 = Matrix Size(0:w359) -> (2:w360:i32)  [unwired: 1 out]
            n175 = Reciprocal(x=w360) -> (1/x=w361:dbl)
            n176 = Initialize Array(w361, w360) -> (w358:dbl[])
            n177 = call-poly <vilib>:"A x B.vi"("Vector"=w358, "A"=w359) -> ("A x Vector"=w357:dbl[])  [unwired: 1 out]
            n178 = Bundle("Wavlength"=w367, "A x Vector"=w357) -> (w369:T11)  [unwired: 1 in]
            n179 = Build Array(w369) -> (w366:T12)
            n180 = property on="XY Graph" class="XYGraph (strict)"("Value"=w366) -> ()  [unwired: 2 in, 2 out]
            n181 = Bundle By Name(cluster=w368, "Dark"=w365) -> (w372:T2)
          }
          frame "Set_Ref" {
            # "Averaging"
            n182 = Unbundle By Name(w377) -> ("Wavlength"=w376:dbl[unit][])
            n183 = Unbundle By Name(w394) -> ("Data_Ref"=w381:T9)
            n184 = Index Array(array=w381, index=0) -> (element=w389:T10)
            n185 = Unbundle By Name(w389) -> ("Image"=w388:dbl[][][])
            n186 = Index Array(array=w388, index (dim 1)=0 ("disabled index (row)")) -> (element=w386:dbl[][])  [unwired: 2 in]
            n187 = Transpose 2D Array(2D array=w386) -> (transposed array=w383:dbl[][])
            n188 = Matrix Size(0:w383) -> (2:w384:i32)  [unwired: 1 out]
            n189 = Reciprocal(x=w384) -> (1/x=w385:dbl)
            n190 = Initialize Array(w385, w384) -> (w382:dbl[])
            n191 = call-poly <vilib>:"A x B.vi"("Vector"=w382, "A"=w383) -> ("A x Vector"=w378:dbl[])  [unwired: 1 out]
            n192 = Bundle("Wavlength"=w376, "A x Vector"=w378) -> (w380:T11)  [unwired: 1 in]
            n193 = Build Array(w380) -> (w379:T12)
            n194 = Bundle By Name(cluster=w377, "Ref"=w381) -> (w391:T2)
            n195 = property on="XY Graph" class="XYGraph (strict)"("Value"=w379) -> ()  [unwired: 2 in, 2 out]
          }
          frame "Set_Wavelength" {
            n196 = Unbundle By Name(w397) -> ("Wavelength"=w400:dbl[unit][])
            n197 = Bundle By Name(cluster=w399, "Wavlength"=w400) -> (w398:T2)
          }
          frame "Spectrometer_Preview" {
            w405 = 0 ("index (page)")
            n198 = Unbundle By Name(w411) -> ("Data_Raw"=w409:T9)
            n199 = Unbundle By Name(w410) -> ("Wavlength"=w404:dbl[unit][])
            n200 = Index Array(array=w409, index=0) -> (element=w407:T10)
            n201 = Unbundle By Name(w407) -> ("Image"=w406:dbl[][][])
            n202 = Index Array(array=w406, index (dim 0)=w405, index (dim 1)=w405) -> (element=w403:dbl[])  [unwired: 1 in]
            n203 = Bundle("Wavlength"=w404, "Image"=w403) -> (w402:cluster{"Wavlength":dbl[unit][], "Image":dbl[]})  [unwired: 1 in]
            n204 = Build Array(w402) -> (→"XY Graph":T1)
          }
        }
      }
      frame Error {
        w419 = T14 4 items=["no dialog", "OK message", "continue or stop message", "OK message + warnings", "continue/stop + warnings"] ("type of dialog (OK msg:1)")
        n205 = call <vilib>:"General Error Handler.vi"("type of dialog (OK msg:1)"=w419, "error in (no error)"=w416) -> ("error out"=w418:errorcluster)  [unwired: 9 in, 4 out]
        n206 = call <vilib>:"Clear Errors.vi"("error in (no error)"=w418) -> ("error out"=w415:errorcluster)  [unwired: 5 in, 1 out]
      }
    }
  }
  n207 = while {
    shift-right: [w422] -> _
    shift-left: w12 -> [w420]
    shift-right: [w425] -> _
    shift-left: w7 -> [w426]
    shift-right: [w423] -> _
    shift-left: w8 -> [w424]
    stop <- w421 stop-if-true
    # "Producer"
    n208 = event shown="[6] \"Integration Time\": Value Change" {
      selector: _ -> [_ _ _ _ _ _ _ _ _ _ _ _ _ _ _ _ _ _ _ _ _]
      dyn-events: _ -> [_ _ _ _ _ _ _ _ _ _ _ _ _ _ _ _ _ _ _ _ _]
      timeout: -1 -> [_ _ _ _ _ _ _ _ _ _ _ _ _ _ _ _ _ _ _ _ _]
      tunnel: w426 -> [w429 w444 w448 w460 w473 w488 w500 w511 w514 w521 w540 w547 w556 w564 w579 w589 w598 w606 w611 w618 w630]
      tunnel: [w429 w441 w448 w460 w473 w488 w500 w511 w514 w521 w540 w547 w556 w563 w579 w589 w598 w606 w611 w616 w630] -> w425
      tunnel: w424 -> [w428 w443 w450 w458 w470 w487 w498 w506 w513 w518 w538 w546 w554 w570 w576 w588 w597 w605 w610 w623 w631]
      tunnel: [w428 w437 w447 w454 w469 w485 w496 w505 w513 w516 w537 w544 w553 w562 w577 w585 w594 w605 w610 w623 w631] -> w423
      tunnel: w420 -> [w430 w445 w451 w459 w472 w489 w499 w508 w515 w519 w541 w548 w557 w572 w580 w590 w599 w607 w612 w624 w629]
      tunnel: [w430 w442 w449 w455 w471 w486 w497 w507 w515 w520 w539 w545 w555 w571 w578 w586 w595 w607 w609 w622 w629] -> w422
      tunnel: [_ TRUE _ _ _ _ _ _ _ _ _ _ _ _ _ _ _ _ _ _ _] -> w421
      event Timeout {
        n209 = event-data() -> ()  [unwired: 1 in, 3 out]
      }
      event "Stop Button": Value Change {
        w433 = T4 {"QueueAction"=enum."TimeOut", "Data"=[], "Data_Raw"=[], "Data_Dark"=[], "Data_Ref"=[], "Device Information"=[], "Numeric Control"=0.0, "Boolean"=FALSE, "Wavelength"=[], "Time"=[], "Time Stamp"=timestamp(0 s since 1904-01-01), "Numeric Control 2"=0.0}  # DataQueue
        w436 = T6 {"QueueAction"=enum."TimeOut", "Numeric 1"=0.0, "Numeric 2"=0.0, "Boolean 1"=FALSE, "Boolean 2"=FALSE, "Spin Program"=[]}  # Device Queue
        n210 = event-data() -> ()  [unwired: 1 in, 6 out]
        n211 = Bundle By Name(cluster=w436, "QueueAction"=DeviceQueue_Action."Close_Program") -> (w434:T6)
        n212 = Enqueue Element(queue=w445, element=w434, error in (no error)=w443) -> (queue out=w442:refnum<queue>, error out=w438:errorcluster)  [unwired: 1 in, 1 out]
        n213 = Bundle By Name(cluster=w433, "QueueAction"=DataQueue_Action."Close_Program") -> (w431:T4)
        n214 = Enqueue Element(queue=w444, element=w431, error in (no error)=w443) -> (queue out=w441:refnum<queue>, error out=w439:errorcluster)  [unwired: 1 in, 1 out]
        n215 = Merge Errors(w439, w438) -> (w437:errorcluster)
      }
      event "Abort Button": Value Change {
        w453 = T6 {"QueueAction"=enum."TimeOut", "Numeric 1"=0.0, "Numeric 2"=0.0, "Boolean 1"=FALSE, "Boolean 2"=FALSE, "Spin Program"=[]}  # Device Queue
        # "At the moment just spin coater in non in-situ measurements can be stopped"
        n216 = event-data() -> ()  [unwired: 1 in, 6 out]
        n217 = Bundle By Name(cluster=w453, "QueueAction"=DeviceQueue_Action."Abort") -> (w452:T6)
        n218 = Enqueue Element(queue=w451, element=w452, error in (no error)=w450) -> (queue out=w449:refnum<queue>, error out=w447:errorcluster)  [unwired: 1 in, 1 out]
      }
      event "Init_Spectrometer": Value Change {
        n219 = event-data() -> ()  [unwired: 1 in, 6 out]
        n220 = case shown="True" "Init_Spectrometer" {
          tunnel: [w461 w464] -> w456
          frame True {
            n221 = Bundle By Name(cluster=T6 {"QueueAction"=enum."TimeOut", "Numeric 1"=0.0, "Numeric 2"=0.0, "Boolean 1"=FALSE, "Boolean 2"=FALSE, "Spin Program"=[]} ("element"), "QueueAction"=DeviceQueue_Action."Spectrometer_Init") -> (w461:T6)
          }
          frame False {
            n222 = Bundle By Name(cluster=T6 {"QueueAction"=enum."TimeOut", "Numeric 1"=0.0, "Numeric 2"=0.0, "Boolean 1"=FALSE, "Boolean 2"=FALSE, "Spin Program"=[]} ("element"), "QueueAction"=DeviceQueue_Action."Spectrometer_Close") -> (w464:T6)
          }
        }
        n223 = Enqueue Element(queue=w459, element=w456, error in (no error)=w458) -> (queue out=w455:refnum<queue>, error out=w454:errorcluster)  [unwired: 1 in, 1 out]
      }
      event "Init_Arduino": Value Change {
        n224 = event-data() -> ("NewVal"=w468:bool)  [unwired: 1 in, 5 out]
        n225 = case shown="True" w468 {
          tunnel: [w474 w477] -> w467
          frame False {
            w476 = T6 {"QueueAction"=enum."TimeOut", "Numeric 1"=0.0, "Numeric 2"=0.0, "Boolean 1"=FALSE, "Boolean 2"=FALSE, "Spin Program"=[]}  # Device Queue
            n226 = Bundle By Name(cluster=w476, "QueueAction"=DeviceQueue_Action."Arduino_Close") -> (w474:T6)
          }
          frame True {
            w479 = T6 {"QueueAction"=enum."TimeOut", "Numeric 1"=0.0, "Numeric 2"=0.0, "Boolean 1"=FALSE, "Boolean 2"=FALSE, "Spin Program"=[]}  # Device Queue
            n227 = Bundle By Name(cluster=w479, "QueueAction"=DeviceQueue_Action."Arduino_Init") -> (w477:T6)
          }
        }
        n228 = Enqueue Element(queue=w472, element=w467, error in (no error)=w470) -> (queue out=w471:refnum<queue>, error out=w469:errorcluster)  [unwired: 1 in, 1 out]
      }
      event "Program Spin Coater\nSpeed (rpm)          Time (s)": Value Change {
        w491 = T6 {"QueueAction"=enum."TimeOut", "Numeric 1"=0.0, "Numeric 2"=0.0, "Boolean 1"=FALSE, "Boolean 2"=FALSE, "Spin Program"=[]}  # Device Queue
        n229 = event-data() -> ("NewVal"=w483:dbl[][])  [unwired: 1 in, 5 out]
        n230 = property on="Seconds to Spin Start" class="DigNum (strict)"() -> ("Value"=w481:dbl[unit])  [unwired: 2 in, 2 out]
        n231 = node(w481) -> (w480:dbl)
        n232 = Bundle By Name(cluster=w491, "QueueAction"=DeviceQueue_Action."Arduino_LoadProgram", "Spin Program"=w483, "Numeric 1"=w480) -> (w490:T6)
        n233 = Enqueue Element(queue=w489, element=w490, error in (no error)=w487) -> (queue out=w486:refnum<queue>, error out=w485:errorcluster)  [unwired: 1 in, 1 out]
        n234 = property on="Integration Time" class="DigNum (strict)"() -> ("Value"=w482:dbl[unit])  [unwired: 2 in, 2 out]
        n235 = property on="Integration Time" class="DigNum (strict)"("Val(Sgnl)"=w482) -> ()  [unwired: 2 in, 2 out]
      }
      event "Integration Time": Value Change {
        w502 = T6 {"QueueAction"=enum."TimeOut", "Numeric 1"=0.0, "Numeric 2"=0.0, "Boolean 1"=FALSE, "Boolean 2"=FALSE, "Spin Program"=[]}  # Device Queue
        n236 = event-data() -> ("NewVal"=w494:dbl[unit])  [unwired: 1 in, 5 out]
        n237 = node(w494) -> (w493:dbl)
        n238 = property on="Calculate Frames" class="Bool (strict)"() -> ("Value"=w492:bool)  [unwired: 2 in, 2 out]
        n239 = Bundle By Name(cluster=w502, "QueueAction"=DeviceQueue_Action."Spectrometer_SetIntegrationTime", "Numeric 1"=w493, "Boolean 1"=w492) -> (w501:T6)
        n240 = Enqueue Element(queue=w499, element=w501, error in (no error)=w498) -> (queue out=w497:refnum<queue>, error out=w496:errorcluster)  [unwired: 1 in, 1 out]
      }
      event "Frames": Value Change {
        w510 = T6 {"QueueAction"=enum."TimeOut", "Numeric 1"=0.0, "Numeric 2"=0.0, "Boolean 1"=FALSE, "Boolean 2"=FALSE, "Spin Program"=[]}  # Device Queue
        n241 = event-data() -> ()  [unwired: 1 in, 6 out]
        n242 = Bundle By Name(cluster=w510, "QueueAction"=DeviceQueue_Action."Spectrometer_SetFrames", "Numeric 1"="Frames") -> (w509:T6)
        n243 = Enqueue Element(queue=w508, element=w509, error in (no error)=w506) -> (queue out=w507:refnum<queue>, error out=w505:errorcluster)  [unwired: 1 in, 1 out]
      }
      event "Seconds to Spin Start", "Seconds after Spin Stop": Value Change {
        n244 = event-data() -> ()  [unwired: 1 in, 6 out]
        n245 = property on="Program Spin Coater\nSpeed (rpm)          Time (s)" class="Arr (strict)"() -> ("Value"=w512:dbl[][])  [unwired: 2 in, 2 out]
        n246 = property on="Program Spin Coater\nSpeed (rpm)          Time (s)" class="Arr (strict)"("Val(Sgnl)"=w512) -> ()  [unwired: 2 in, 2 out]
      }
      event "Calculate Frames": Value Change {
        n247 = event-data() -> ("NewVal"=w522:bool)  [unwired: 1 in, 5 out]
        n248 = case shown="False" w522 {
          tunnel: [0 2] -> w517
          tunnel: w519 -> [w524 w533]
          tunnel: [w524 w531] -> w520
          tunnel: w518 -> [w523 w530]
          tunnel: [w523 w526] -> w516
          frame False {
          }
          frame True {
            w532 = T6 {"QueueAction"=enum."TimeOut", "Numeric 1"=0.0, "Numeric 2"=0.0, "Boolean 1"=FALSE, "Boolean 2"=FALSE, "Spin Program"=[]}  # Device Queue
            n249 = property on="Integration Time" class="DigNum (strict)"() -> ("Value"=w528:dbl[unit])  [unwired: 2 in, 2 out]
            n250 = node(w528) -> (w527:dbl)
            n251 = Bundle By Name(cluster=w532, "QueueAction"=DeviceQueue_Action."Spectrometer_SetIntegrationTime", "Numeric 1"=w527) -> (w534:T6)
            n252 = Enqueue Element(queue=w533, element=w534, error in (no error)=w530) -> (queue out=w531:refnum<queue>, error out=w526:errorcluster)  [unwired: 1 in, 1 out]
          }
        }
        n253 = property on="Frames" class="DigNum (strict)"("DisabledEnum"=w517) -> ()  [unwired: 2 in, 2 out]
      }
      event "Record RefSpec": Value Change {
        w543 = T6 {"QueueAction"=enum."TimeOut", "Numeric 1"=0.0, "Numeric 2"=0.0, "Boolean 1"=FALSE, "Boolean 2"=FALSE, "Spin Program"=[]}  # Device Queue
        n254 = event-data() -> ()  [unwired: 1 in, 6 out]
        n255 = Bundle By Name(cluster=w543, "QueueAction"=DeviceQueue_Action."Spectrometer_SetReference") -> (w542:T6)
        n256 = Enqueue Element(queue=w541, element=w542, error in (no error)=w538) -> (queue out=w539:refnum<queue>, error out=w537:errorcluster)  [unwired: 1 in, 1 out]
      }
      event "Preview": Value Change {
        w551 = T6 {"QueueAction"=enum."TimeOut", "Numeric 1"=0.0, "Numeric 2"=0.0, "Boolean 1"=FALSE, "Boolean 2"=FALSE, "Spin Program"=[]}  # Device Queue
        n257 = event-data() -> ()  [unwired: 1 in, 6 out]
        n258 = Bundle By Name(cluster=w551, "QueueAction"=DeviceQueue_Action."Spectrometer_Preview") -> (w550:T6)
        n259 = Enqueue Element(queue=w548, element=w550, error in (no error)=w546) -> (queue out=w545:refnum<queue>, error out=w544:errorcluster)  [unwired: 1 in, 1 out]
      }
      event "Record_Darkspec": Value Change {
        w559 = T6 {"QueueAction"=enum."TimeOut", "Numeric 1"=0.0, "Numeric 2"=0.0, "Boolean 1"=FALSE, "Boolean 2"=FALSE, "Spin Program"=[]}  # Device Queue
        n260 = event-data() -> ()  [unwired: 1 in, 6 out]
        n261 = Bundle By Name(cluster=w559, "QueueAction"=DeviceQueue_Action."Spectrometer_SetDarkspec") -> (w558:T6)
        n262 = Enqueue Element(queue=w557, element=w558, error in (no error)=w554) -> (queue out=w555:refnum<queue>, error out=w553:errorcluster)  [unwired: 1 in, 1 out]
      }
      event "StartMeasurement_Button": Value Change {
        w566 = T4 {"QueueAction"=enum."TimeOut", "Data"=[], "Data_Raw"=[], "Data_Dark"=[], "Data_Ref"=[], "Device Information"=[], "Numeric Control"=0.0, "Boolean"=FALSE, "Wavelength"=[], "Time"=[], "Time Stamp"=timestamp(0 s since 1904-01-01), "Numeric Control 2"=0.0}  # DataQueue
        w574 = T6 {"QueueAction"=enum."TimeOut", "Numeric 1"=0.0, "Numeric 2"=0.0, "Boolean 1"=FALSE, "Boolean 2"=FALSE, "Spin Program"=[]}  # Device Queue
        n263 = event-data() -> ()  [unwired: 1 in, 6 out]
        n264 = property on="Preview" class="Bool (strict)"("Value"=FALSE ("Preview")) -> ()  [unwired: 2 in, 2 out]
        n265 = Bundle By Name(cluster=w574, "QueueAction"=DeviceQueue_Action."Measure_InSitu") -> (w573:T6)
        n266 = Enqueue Element(queue=w572, element=w573, error in (no error)=w570) -> (queue out=w571:refnum<queue>, error out=w561:errorcluster)  [unwired: 1 in, 1 out]
        n267 = Get Date/Time In Seconds() -> (seconds since 1Jan1904=w560:timestamp)
        n268 = Bundle By Name(cluster=w566, "QueueAction"=DataQueue_Action."Measure_InSituSpinCoating", "Time Stamp"=w560) -> (w567:T4)
        n269 = Enqueue Element(queue=w564, element=w567, error in (no error)=w561) -> (queue out=w563:refnum<queue>, error out=w562:errorcluster)  [unwired: 1 in, 1 out]
      }
      event "StartSpin_Button": Value Change {
        w582 = T6 {"QueueAction"=enum."TimeOut", "Numeric 1"=0.0, "Numeric 2"=0.0, "Boolean 1"=FALSE, "Boolean 2"=FALSE, "Spin Program"=[]}  # Device Queue
        n270 = event-data() -> ()  [unwired: 1 in, 6 out]
        n271 = Bundle By Name(cluster=w582, "QueueAction"=DeviceQueue_Action."Arduino_StartProgram") -> (w581:T6)
        n272 = Enqueue Element(queue=w580, element=w581, error in (no error)=w576) -> (queue out=w578:refnum<queue>, error out=w577:errorcluster)  [unwired: 1 in, 1 out]
      }
      event "Milliseconds": Value Change {
        w591 = T6 {"QueueAction"=enum."TimeOut", "Numeric 1"=0.0, "Numeric 2"=0.0, "Boolean 1"=FALSE, "Boolean 2"=FALSE, "Spin Program"=[]}  # Device Queue
        n273 = event-data() -> ()  [unwired: 1 in, 6 out]
        n274 = Bundle By Name(cluster=w591, "QueueAction"=DeviceQueue_Action."Arduino_SetMillis", "Numeric 1"="Milliseconds") -> (w587:T6)
        n275 = Enqueue Element(queue=w590, element=w587, error in (no error)=w588) -> (queue out=w586:refnum<queue>, error out=w585:errorcluster)  [unwired: 1 in, 1 out]
      }
      event "Speed": Value Change {
        w600 = T6 {"QueueAction"=enum."TimeOut", "Numeric 1"=0.0, "Numeric 2"=0.0, "Boolean 1"=FALSE, "Boolean 2"=FALSE, "Spin Program"=[]}  # Device Queue
        n276 = event-data() -> ()  [unwired: 1 in, 6 out]
        n277 = Bundle By Name(cluster=w600, "QueueAction"=DeviceQueue_Action."Arduino_SetSpeed", "Numeric 1"="Speed") -> (w596:T6)
        n278 = Enqueue Element(queue=w599, element=w596, error in (no error)=w597) -> (queue out=w595:refnum<queue>, error out=w594:errorcluster)  [unwired: 1 in, 1 out]
      }
      event "Debug": Value Change {
        n279 = event-data() -> ()  [unwired: 1 in, 6 out]
        n280 = Select(t=u8 0, s="Debug", f=u8 2) -> (s? t:f=w601:u8)
        n281 = property on="Milliseconds" class="DigNum (strict)"("DisabledEnum"=w601) -> ()  [unwired: 2 in, 2 out]
        n282 = property on="Speed" class="DigNum (strict)"("DisabledEnum"=w601) -> ()  [unwired: 2 in, 2 out]
      }
      event "Frames for Spectrometer": Value Change {
        w614 = T6 {"QueueAction"=enum."TimeOut", "Numeric 1"=0.0, "Numeric 2"=0.0, "Boolean 1"=FALSE, "Boolean 2"=FALSE, "Spin Program"=[]}  # Device Queue
        n283 = event-data() -> ("NewVal"=w608:dbl)  [unwired: 1 in, 5 out]
        n284 = Bundle By Name(cluster=w614, "QueueAction"=DeviceQueue_Action."Spectrometer_SetFrames", "Numeric 1"=w608) -> (w615:T6)
        n285 = Enqueue Element(queue=w612, element=w615) -> (queue out=w609:refnum<queue>)  [unwired: 2 in, 2 out]
      }
      event "Measure Spectrum": Value Change {
        w620 = T4 {"QueueAction"=enum."TimeOut", "Data"=[], "Data_Raw"=[], "Data_Dark"=[], "Data_Ref"=[], "Device Information"=[], "Numeric Control"=0.0, "Boolean"=FALSE, "Wavelength"=[], "Time"=[], "Time Stamp"=timestamp(0 s since 1904-01-01), "Numeric Control 2"=0.0}  # DataQueue
        w626 = T6 {"QueueAction"=enum."TimeOut", "Numeric 1"=0.0, "Numeric 2"=0.0, "Boolean 1"=FALSE, "Boolean 2"=FALSE, "Spin Program"=[]}  # Device Queue
        n286 = event-data() -> ()  [unwired: 1 in, 6 out]
        n287 = Bundle By Name(cluster=w626, "QueueAction"=DeviceQueue_Action."Measure_Spectrum") -> (w627:T6)
        n288 = Enqueue Element(queue=w624, element=w627) -> (queue out=w622:refnum<queue>)  [unwired: 2 in, 2 out]
        n289 = Get Date/Time In Seconds() -> (seconds since 1Jan1904=w621:timestamp)
        n290 = Bundle By Name(cluster=w620, "QueueAction"=DataQueue_Action."Measure_Spectrum", "Time Stamp"=w621) -> (w617:T4)
        n291 = Enqueue Element(queue=w618, element=w617) -> (queue out=w616:refnum<queue>)  [unwired: 2 in, 2 out]
      }
      event "Automatically \nadjust count": Value Change {
        n292 = event-data() -> ("NewVal"=w634:bool)  [unwired: 1 in, 5 out]
        n293 = Select(t=u8 2, s=w634, f=u8 0) -> (s? t:f=w628:u8)
        n294 = property on="Spectra Count" class="DigNum (strict)"("DisabledEnum"=w628) -> ()  [unwired: 2 in, 2 out]
      }
    }
  }
  n295 = while {
    shift-right: [w639] -> _
    shift-left: w8 -> [w643]
    shift-right: [w640] -> w10
    shift-left: w12 -> [w642]
    shift-right: [w637] -> w9
    shift-left: w7 -> [w638]
    shift-right: [w635] -> _
    shift-left: w11 -> [w636]
    stop <- w641 stop-if-true
    # "Consumer Devices"
    n296 = case shown="No Error" w643 {
      selector: w643 -> [w655 w1063]
      tunnel: w642 -> [w656 w1064]
      tunnel: [w652 _] -> w641
      tunnel: [w651 w1064] -> w640
      tunnel: [w649 w1060] -> w639
      tunnel: w638 -> [w647 w1058]
      tunnel: [w648 w1058] -> w637
      tunnel: w636 -> [w646 w1059]
      tunnel: [w645 w1059] -> w635
      frame No Error {
        n297 = Dequeue Element(queue=w656, error in (no error)=w655) -> (queue out=w654:refnum<queue>, element=w644:T6, error out=w650:errorcluster)  [unwired: 1 in, 1 out]
        n298 = Unbundle By Name(w644) -> ("QueueAction"=w653:T7)
        n299 = case shown="\"Measure_InSitu\"" w653 {
          tunnel: w654 -> [w660 w680 w686 w695 w745 w759 w769 w788 w795 w814 w815 w843 w860 w875 w885 w897 w909 w922 w942 w944 w951 w967 w980 w990 w1036 w1055]
          tunnel: [_ w682 _ _ _ _ _ _ _ _ _ _ _ _ _ _ _ _ _ _ _ _ _ _ _ _] -> w652
          tunnel: [w660 w665 w686 w694 w745 w759 w770 w788 w795 w814 w815 w843 w860 w875 w885 w897 w902 w922 w942 w944 w951 w967 w980 w990 w998 w1046] -> w651
          tunnel: w650 -> [w659 w664 w687 w706 w746 w758 w765 w791 w799 w811 w825 w841 w850 w866 w882 w893 w917 w926 w941 w946 w958 w968 w979 w983 w992 w1054]
          tunnel: [w659 w663 w685 w693 w740 w757 w763 w789 w796 w801 w819 w840 w847 w862 w880 w887 w901 w925 w937 w945 w952 w966 w975 w982 w999 w1045] -> w649
          tunnel: [w657 w662 w690 w691 w742 w754 w774 w787 w794 w805 w827 w844 w854 w869 w876 w889 w915 w924 w939 w950 w962 w964 w981 w985 w1007 w1053] -> w648
          tunnel: w647 -> [w657 w662 w690 w692 w742 w755 w775 w787 w794 w806 w827 w844 w857 w872 w876 w891 w915 w924 w939 w950 w962 w964 w981 w986 w1007 w1053]
          tunnel: w646 -> [w658 w661 w689 w703 w744 w756 w768 w786 w798 w807 w818 w837 w853 w868 w879 w886 w914 w923 w938 w949 w961 w963 w978 w984 w1039 w1052]
          tunnel: [w658 w661 w689 w697 w743 w756 w767 w784 w793 w807 w816 w838 w852 w867 w877 w886 w912 w923 w938 w949 w961 w963 w978 w984 w1039 w1052] -> w645
          tunnel: w644 -> [_ _ _ _ _ _ _ _ _ w813 w822 w845 _ _ w883 _ _ _ w936 _ w959 w965 _ _ _ _]
          frame "TimeOut", Default {
          }
          frame "Close_Program" {
            w681 = T6 {"QueueAction"=enum."TimeOut", "Numeric 1"=0.0, "Numeric 2"=0.0, "Boolean 1"=FALSE, "Boolean 2"=FALSE, "Spin Program"=[]}  # Device Queue
            n300 = Bundle By Name(cluster=w681, "QueueAction"=DeviceQueue_Action."Spectrometer_Close") -> (w676:T6)
            n301 = Bundle By Name(cluster=w676, "QueueAction"=DeviceQueue_Action."Laser_Close") -> (w674:T6)
            n302 = Bundle By Name(cluster=w674, "QueueAction"=DeviceQueue_Action."Arduino_Close") -> (w668:T6)
            n303 = Enqueue Element(queue=w680, element=w676, error in (no error)=w664) -> (queue out=w678:refnum<queue>, error out=w673:errorcluster)  [unwired: 1 in, 1 out]
            n304 = Bundle By Name(cluster=w668, "QueueAction"=DeviceQueue_Action."Close_Program") -> (w666:T6)
            n305 = Enqueue Element(queue=w678, element=w674, error in (no error)=w673) -> (queue out=w672:refnum<queue>, error out=w671:errorcluster)  [unwired: 1 in, 1 out]
            n306 = Enqueue Element(queue=w672, element=w668, error in (no error)=w671) -> (queue out=w670:refnum<queue>, error out=w669:errorcluster)  [unwired: 1 in, 1 out]
            n307 = Enqueue Element(queue=w670, element=w666, error in (no error)=w669) -> (queue out=w665:refnum<queue>, error out=w663:errorcluster)  [unwired: 1 in, 1 out]
            n308 = First Call?() -> (First Call?: T/F=w683:bool)
            n309 = Not(x=w683) -> (.not. x?=w682:bool)
          }
          frame "Abort" {
            n310 = Unbundle By Name(w689) -> ("Port Arduino"=w688:refnum<visa-resource-name>)
            n311 = VISA Write(VISA resource name=w688, write buffer="abo", error in (no error)=w687) -> (error out=w685:errorcluster)  [unwired: 2 out]
          }
          frame "Spectrometer_Init" {
            n312 = call-dynamic "Init.vi"("error in (no error)"=w706, "Variant"=0, "Avantes in"=refnum<class "Avantes.lvclass"> refnum ("Avantes.lvclass")) -> ("error out"=w705:errorcluster, "Avantes out"=w704:refnum<class "Avantes.lvclass">)  [unwired: 7 in]
            n313 = call-dynamic "IsInit.vi"("error in (no error)"=w705, "Avantes in"=w704) -> ("error out"=w701:errorcluster, "Is Init?"=w700:bool, "Avantes out"=w702:refnum<class "Avantes.lvclass">)  [unwired: 7 in]
            n314 = property on="Spectromter" class="Bool (strict)"("Value"=w700) -> ()  [unwired: 2 in, 2 out]
            n315 = property on="Init_Spectrometer" class="Bool (strict)"("Value"=w700) -> ()  [unwired: 2 in, 2 out]
            n316 = call-dynamic "Set_ExposurePerFrame.vi"("error in (no error)"=w701, "Exposure per Frame"=1, "Avantes in"=w702) -> ("error out"=w696:errorcluster, "Avantes out"=w699:refnum<class "Avantes.lvclass">)  [unwired: 7 in]
            n317 = case shown="True" w700 {
              tunnel: w699 -> [_ w722]
              tunnel: w696 -> [w711 w720]
              tunnel: [refnum<class "Abstract_CCD.lvclass"> refnum ("Abstract_CCD.lvclass") w721] -> w698
              tunnel: w695 -> [w712 w737]
              tunnel: [w712 w726] -> w694
              tunnel: [w711 w725] -> w693
              tunnel: w692 -> [w710 w717]
              tunnel: [w710 w715] -> w691
              frame False {
              }
              frame True {
                w723 = T4 {"QueueAction"=enum."TimeOut", "Data"=[], "Data_Raw"=[], "Data_Dark"=[], "Data_Ref"=[], "Device Information"=[], "Numeric Control"=0.0, "Boolean"=FALSE, "Wavelength"=[], "Time"=[], "Time Stamp"=timestamp(0 s since 1904-01-01), "Numeric Control 2"=0.0}  # DataQueue
                w738 = T6 {"QueueAction"=enum."TimeOut", "Numeric 1"=0.0, "Numeric 2"=0.0, "Boolean 1"=FALSE, "Boolean 2"=FALSE, "Spin Program"=[]}  # Device Queue
                n318 = call-dynamic "Get_WavelengthAxis.vi"("error in (no error)"=w720, "Avantes in"=w722) -> ("error out"=w719:errorcluster, "lambda"=w714:dbl[unit][], "Avantes out"=w721:refnum<class "Avantes.lvclass">)  [unwired: 7 in]
                n319 = property on="Calculate Frames" class="Bool (strict)"() -> ("Value"=w730:bool)  [unwired: 2 in, 2 out]
                n320 = property on="Integration Time" class="DigNum (strict)"() -> ("Value"=w735:dbl[unit])  [unwired: 2 in, 2 out]
                n321 = Unbundle(w719) -> ("status"=w718:bool)  [unwired: 2 out]
                n322 = node(w735) -> (w734:dbl)
                n323 = Bundle By Name(cluster=w738, "QueueAction"=DeviceQueue_Action."Spectrometer_SetIntegrationTime", "Numeric 1"=w734, "Boolean 1"=w730) -> (w732:T6)
                n324 = property on="Frames" class="DigNum (strict)"() -> ("Value"=w729:i32)  [unwired: 2 in, 2 out]
                n325 = property on="Error_Spectromter" class="Bool (strict)"("Value"=w718) -> ()  [unwired: 2 in, 2 out]
                n326 = Enqueue Element(queue=w737, element=w732, error in (no error)=w720) -> (queue out=w733:refnum<queue>, error out=w727:errorcluster)  [unwired: 1 in, 1 out]
                n327 = Bundle By Name(cluster=w732, "QueueAction"=DeviceQueue_Action."Spectrometer_SetFrames", "Numeric 1"=w729) -> (w728:T6)
                n328 = Bundle By Name(cluster=w723, "QueueAction"=DataQueue_Action."Set_Wavelength", "Wavelength"=w714) -> (w724:T4)
                n329 = Enqueue Element(queue=w717, element=w724) -> (queue out=w715:refnum<queue>)  [unwired: 2 in, 2 out]
                n330 = Enqueue Element(queue=w733, element=w728, error in (no error)=w727) -> (queue out=w726:refnum<queue>, error out=w725:errorcluster)  [unwired: 1 in, 1 out]
              }
            }
            n331 = Bundle By Name(cluster=w703, "Abstract_CCD.lvclass"=w698) -> (w697:T3)
          }
          frame "Spectrometer_Close" {
            n332 = property on="Spectromter" class="Bool (strict)"("Value"=FALSE ("Spectromter")) -> ()  [unwired: 2 in, 2 out]
            n333 = Unbundle By Name(w744) -> ("Abstract_CCD.lvclass"=w747:refnum<class "Abstract_CCD.lvclass">)
            n334 = flat-sequence {
              tunnel: [refnum<class "Abstract_CCD.lvclass"> refnum ("Abstract_CCD.lvclass")] -> w741
              tunnel: w740 -> [_]
              frame #0 {
              }
            }
            n335 = call-dynamic "Close.vi"("error in (no error)"=w746, "Abstract_CCD in"=w747) -> ("error out"=w740:errorcluster)  [unwired: 8 in, 1 out]
            n336 = Bundle By Name(cluster=w744, "Abstract_CCD.lvclass"=w741) -> (w743:T3)
          }
          frame "Spectrometer_Measure" {
            w761 = T4 {"QueueAction"=enum."TimeOut", "Data"=[], "Data_Raw"=[], "Data_Dark"=[], "Data_Ref"=[], "Device Information"=[], "Numeric Control"=0.0, "Boolean"=FALSE, "Wavelength"=[], "Time"=[], "Time Stamp"=timestamp(0 s since 1904-01-01), "Numeric Control 2"=0.0}  # DataQueue
            n337 = Unbundle By Name(w756) -> ("Abstract_CCD.lvclass"=w760:refnum<class "Abstract_CCD.lvclass">)
            n338 = call-dynamic "Measure.vi"("error in (no error)"=w758, "Abstract_CCD in"=w760) -> ("error out"=w757:errorcluster, "Data Raw"=w751:T9, "Data"=w752:T9, "Darkspec"=w750:T9, "Time"=w749:dbl[])  [unwired: 3 in, 2 out]
            n339 = Bundle By Name(cluster=w761, "QueueAction"=DataQueue_Action."Spectrometer_Measure", "Data"=w752, "Data_Raw"=w751, "Data_Dark"=w750, "Time"=w749) -> (w762:T4)
            n340 = Enqueue Element(queue=w755, element=w762) -> (queue out=w754:refnum<queue>)  [unwired: 2 in, 2 out]
          }
          frame "Spectrometer_Preview" {
            w776 = T4 {"QueueAction"=enum."TimeOut", "Data"=[], "Data_Raw"=[], "Data_Dark"=[], "Data_Ref"=[], "Device Information"=[], "Numeric Control"=0.0, "Boolean"=FALSE, "Wavelength"=[], "Time"=[], "Time Stamp"=timestamp(0 s since 1904-01-01), "Numeric Control 2"=0.0}  # DataQueue
            n341 = Unbundle By Name(w768) -> ("Abstract_CCD.lvclass"=w766:refnum<class "Abstract_CCD.lvclass">)
            n342 = call-dynamic "Measure.vi"("error in (no error)"=w765, "Abstract_CCD in"=w766) -> ("error out"=w763:errorcluster, "Data Raw"=w773:T9, "Abstract_CCD out"=w764:refnum<class "Abstract_CCD.lvclass">)  [unwired: 3 in, 4 out]
            n343 = property on="Preview" class="Bool (strict)"(error in=w763) -> ("Value"=w771:bool)  [unwired: 1 in, 2 out]
            n344 = case shown="True" w771 {
              tunnel: [w778 w780] -> w770
              tunnel: w769 -> [w778 w779]
              frame False {
              }
              frame True {
                w782 = T6 {"QueueAction"=enum."TimeOut", "Numeric 1"=0.0, "Numeric 2"=0.0, "Boolean 1"=FALSE, "Boolean 2"=FALSE, "Spin Program"=[]}  # Device Queue
                n345 = Bundle By Name(cluster=w782, "QueueAction"=DeviceQueue_Action."Spectrometer_Preview") -> (w781:T6)
                n346 = Enqueue Element(queue=w779, element=w781) -> (queue out=w780:refnum<queue>)  [unwired: 2 in, 2 out]
              }
            }
            n347 = Bundle By Name(cluster=w776, "Data_Raw"=w773, "QueueAction"=DataQueue_Action."Spectrometer_Preview") -> (w777:T4)
            n348 = Enqueue Element(queue=w775, element=w777) -> (queue out=w774:refnum<queue>)  [unwired: 2 in, 2 out]
            n349 = Bundle By Name(cluster=w768, "Abstract_CCD.lvclass"=w764) -> (w767:T3)
          }
          frame "Spectrometer_StartMeasurement" {
            n350 = Unbundle By Name(w786) -> ("Abstract_CCD.lvclass"=w790:refnum<class "Abstract_CCD.lvclass">)
            n351 = call-dynamic "StartMeasure.vi"("error in (no error)"=w791, "Frames"=-1, "Abstract_CCD in"=w790) -> ("error out"=w789:errorcluster, "Abstract_CCD out"=w785:refnum<class "Abstract_CCD.lvclass">)  [unwired: 7 in]
            n352 = Bundle By Name(cluster=w786, "Abstract_CCD.lvclass"=w785) -> (w784:T3)
          }
          frame "Spectrometer_StopMeasurement" {
            n353 = Unbundle By Name(w798) -> ("Abstract_CCD.lvclass"=w800:refnum<class "Abstract_CCD.lvclass">)
            n354 = call-dynamic "StopMeasurement.vi"("error in (no error)"=w799, "Abstract_CCD in"=w800) -> ("error out"=w796:errorcluster, "Abstract_CCD out"=w797:refnum<class "Abstract_CCD.lvclass">)  [unwired: 8 in]
            n355 = Bundle By Name(cluster=w798, "Abstract_CCD.lvclass"=w797) -> (w793:T3)
          }
          frame "Spectrometer_GetData" {
            w810 = T4 {"QueueAction"=enum."TimeOut", "Data"=[], "Data_Raw"=[], "Data_Dark"=[], "Data_Ref"=[], "Device Information"=[], "Numeric Control"=0.0, "Boolean"=FALSE, "Wavelength"=[], "Time"=[], "Time Stamp"=timestamp(0 s since 1904-01-01), "Numeric Control 2"=0.0}  # DataQueue
            n356 = Unbundle By Name(w807) -> ("Abstract_CCD.lvclass"=w812:refnum<class "Abstract_CCD.lvclass">)
            n357 = Unbundle By Name(w813) -> ("Numeric 1"=w804:dbl)
            n358 = call-dynamic "Measure_GetData.vi"("error in (no error)"=w811, "SpectraCount"=w804, "Abstract_CCD in"=w812) -> ("error out"=w801:errorcluster, "Data_Raw"=w803:T9, "Time"=w802:dbl[])  [unwired: 5 in, 1 out]
            n359 = Bundle By Name(cluster=w810, "QueueAction"=DataQueue_Action."Spectrometer_Measure", "Data_Raw"=w803, "Time"=w802) -> (w809:T4)
            n360 = Enqueue Element(queue=w806, element=w809) -> (queue out=w805:refnum<queue>)  [unwired: 2 in, 2 out]
          }
          frame "Spectrometer_SetIntegrationTime" {
            n361 = Unbundle By Name(w822) -> ("Numeric 1"=w824:dbl)
            n362 = Unbundle By Name(w818) -> ("Abstract_CCD.lvclass"=w826:refnum<class "Abstract_CCD.lvclass">)
            n363 = Unbundle By Name(w822) -> ("Boolean 1"=w821:bool)
            n364 = node(w824) -> (w823:dbl[unit])
            n365 = call-dynamic "Set_ExposureTime.vi"("error in (no error)"=w825, "Exposure Time"=w823, "Abstract_CCD in"=w826) -> ("error out"=w829:errorcluster, "Abstract_CCD out"=w828:refnum<class "Abstract_CCD.lvclass">)  [unwired: 7 in]
            n366 = call-dynamic "Get_FrameRate.vi"("error in (no error)"=w829, "Abstract_CCD in"=w828) -> ("error out"=w819:errorcluster, "Frame Rate"=w820:dbl[unit], "Abstract_CCD out"=w817:refnum<class "Abstract_CCD.lvclass">)  [unwired: 7 in]
            "Frame Rate" <- w820
            n367 = Bundle By Name(cluster=w818, "Abstract_CCD.lvclass"=w817) -> (w816:T3)
            n368 = case shown="True" w821 {
              tunnel: w820 -> [_ w832]
              frame False {
              }
              frame True {
                n369 = property on="Program Spin Coater\nSpeed (rpm)          Time (s)" class="Arr (strict)"() -> ("Value"=w835:dbl[][])  [unwired: 2 in, 2 out]
                n370 = property on="Seconds to Spin Start" class="DigNum (strict)"() -> ("Value"=w834:dbl[unit])  [unwired: 2 in, 2 out]
                n371 = property on="Seconds after Spin Stop" class="DigNum (strict)"() -> ("Value"=w833:dbl[unit])  [unwired: 2 in, 2 out]
                n372 = call "CalculateFrames.vi"("Program Spin Coater\nSpeed (rpm)          Time (s)"=w835, "Seconds End"=w833, "Seconds Start"=w834, "Frame Rate"=w832) -> ("Time"=w831:dbl, "Frames"=w830:i32)  [unwired: 6 in]
                n373 = property on="Overall Time" class="DigNum (strict)"("Value"=w831) -> ()  [unwired: 2 in, 2 out]
                n374 = property on="Frames" class="DigNum (strict)"("Value"=w830) -> ()  [unwired: 2 in, 2 out]
              }
            }
          }
          frame "Spectrometer_SetFrames" {
            n375 = Unbundle By Name(w837) -> ("Abstract_CCD.lvclass"=w842:refnum<class "Abstract_CCD.lvclass">)
            n376 = Unbundle By Name(w845) -> ("Numeric 1"=w839:dbl)
            n377 = call-dynamic "Set_Frames.vi"("error in (no error)"=w841, "Frames"=w839, "Abstract_CCD in"=w842) -> ("error out"=w840:errorcluster, "Abstract_CCD out"=w836:refnum<class "Abstract_CCD.lvclass">)  [unwired: 7 in]
            n378 = Bundle By Name(cluster=w837, "Abstract_CCD.lvclass"=w836) -> (w838:T3)
          }
          frame "Spectrometer_SetDarkspec" {
            w858 = T4 {"QueueAction"=enum."TimeOut", "Data"=[], "Data_Raw"=[], "Data_Dark"=[], "Data_Ref"=[], "Device Information"=[], "Numeric Control"=0.0, "Boolean"=FALSE, "Wavelength"=[], "Time"=[], "Time Stamp"=timestamp(0 s since 1904-01-01), "Numeric Control 2"=0.0}  # DataQueue
            n379 = Unbundle By Name(w853) -> ("Abstract_CCD.lvclass"=w851:refnum<class "Abstract_CCD.lvclass">)
            n380 = call-dynamic "Measure.vi"("error in (no error)"=w850, "Abstract_CCD in"=w851) -> ("error out"=w848:errorcluster, "Data Raw"=w855:T9, "Abstract_CCD out"=w849:refnum<class "Abstract_CCD.lvclass">)  [unwired: 3 in, 4 out]
            n381 = Bundle By Name(cluster=w858, "QueueAction"=DataQueue_Action."Set_Dark", "Data_Dark"=w855) -> (w859:T4)
            n382 = Enqueue Element(queue=w857, element=w859) -> (queue out=w854:refnum<queue>)  [unwired: 2 in, 2 out]
            n383 = Bundle By Name(cluster=w853, "Abstract_CCD.lvclass"=w849) -> (w852:T3)
            n384 = property on="Record_Darkspec" class="Bool (strict)"(error in=w848, "Value"=FALSE ("Record_Darkspec")) -> (error out=w847:errorcluster)  [unwired: 1 in, 1 out]
          }
          frame "Spectrometer_SetReference" {
            w873 = T4 {"QueueAction"=enum."TimeOut", "Data"=[], "Data_Raw"=[], "Data_Dark"=[], "Data_Ref"=[], "Device Information"=[], "Numeric Control"=0.0, "Boolean"=FALSE, "Wavelength"=[], "Time"=[], "Time Stamp"=timestamp(0 s since 1904-01-01), "Numeric Control 2"=0.0}  # DataQueue
            n385 = Unbundle By Name(w868) -> ("Abstract_CCD.lvclass"=w865:refnum<class "Abstract_CCD.lvclass">)
            n386 = call-dynamic "Measure.vi"("error in (no error)"=w866, "Abstract_CCD in"=w865) -> ("error out"=w863:errorcluster, "Data Raw"=w870:T9, "Abstract_CCD out"=w864:refnum<class "Abstract_CCD.lvclass">)  [unwired: 3 in, 4 out]
            n387 = Bundle By Name(cluster=w873, "QueueAction"=DataQueue_Action."Set_Ref", "Data_Ref"=w870) -> (w874:T4)
            n388 = Enqueue Element(queue=w872, element=w874) -> (queue out=w869:refnum<queue>)  [unwired: 2 in, 2 out]
            n389 = Bundle By Name(cluster=w868, "Abstract_CCD.lvclass"=w864) -> (w867:T3)
            n390 = property on="Record RefSpec" class="Bool (strict)"(error in=w863, "Value"=FALSE ("Record RefSpec")) -> (error out=w862:errorcluster)  [unwired: 1 in, 1 out]
          }
          frame "Spectrometer_SetTriggerMode" {
            n391 = Unbundle By Name(w879) -> ("Abstract_CCD.lvclass"=w884:refnum<class "Abstract_CCD.lvclass">)
            n392 = Unbundle By Name(w883) -> ("Numeric 1"=w881:dbl)
            n393 = call-dynamic "Set_TriggerMode.vi"("error in (no error)"=w882, "Trigger Mode"=w881, "Abstract_CCD in"=w884) -> ("error out"=w880:errorcluster, "Abstract_CCD out"=w878:refnum<class "Abstract_CCD.lvclass">)  [unwired: 7 in]
            n394 = Bundle By Name(cluster=w879, "Abstract_CCD.lvclass"=w878) -> (w877:T3)
          }
          frame "Spectrometer_DeviceInformation" {
            w892 = T4 {"QueueAction"=enum."TimeOut", "Data"=[], "Data_Raw"=[], "Data_Dark"=[], "Data_Ref"=[], "Device Information"=[], "Numeric Control"=0.0, "Boolean"=FALSE, "Wavelength"=[], "Time"=[], "Time Stamp"=timestamp(0 s since 1904-01-01), "Numeric Control 2"=0.0}  # DataQueue
            n395 = Unbundle By Name(w886) -> ("Abstract_CCD.lvclass"=w894:refnum<class "Abstract_CCD.lvclass">)
            n396 = call-dynamic "Get_DeviceInformation.vi"("error in (no error)"=w893, "Abstract_CCD in"=w894) -> ("error out"=w888:errorcluster, "Array"=w895:string[])  [unwired: 7 in, 1 out]
            n397 = Bundle By Name(cluster=w892, "QueueAction"=DataQueue_Action."Transfer_Settings", "Device Information"=w895) -> (w890:T4)
            n398 = Enqueue Element(queue=w891, element=w890, error in (no error)=w888) -> (queue out=w889:refnum<queue>, error out=w887:errorcluster)  [unwired: 1 in, 1 out]
          }
          frame "Arduino_Init" {
            w911 = T6 {"QueueAction"=enum."TimeOut", "Numeric 1"=0.0, "Numeric 2"=0.0, "Boolean 1"=FALSE, "Boolean 2"=FALSE, "Spin Program"=[]}  # Device Queue
            n399 = call-poly "VISA Configure Serial Port"("VISA resource name"="Port Arduino", "baud rate (9600)"=u32 115200, "error in (no error)"=w917) -> ("VISA resource name out"=w913:refnum<visa-resource-name>, "error out"=w900:errorcluster)  [unwired: 11 in]
            n400 = Unbundle(w900) -> ("status"=w899:bool)  [unwired: 2 out]
            n401 = Not(x=w899) -> (.not. x?=w898:bool)
            n402 = property on="Arduino" class="Bool (strict)"("Value"=w898) -> ()  [unwired: 2 in, 2 out]
            n403 = property on="Program Spin Coater\nSpeed (rpm)          Time (s)" class="Arr (strict)"() -> ("Value"=w906:dbl[][])  [unwired: 2 in, 2 out]
            n404 = Bundle By Name(cluster=w911, "QueueAction"=DeviceQueue_Action."Arduino_LoadProgram", "Spin Program"=dbl[][] []) -> (w907:T6)
            n405 = Enqueue Element(queue=w909, element=w907, error in (no error)=w900) -> (queue out=w905:refnum<queue>, error out=w904:errorcluster)  [unwired: 1 in, 1 out]
            n406 = Bundle By Name(cluster=w907, "Spin Program"=w906) -> (w903:T6)
            n407 = Bundle By Name(cluster=w914, "Port Arduino"=w913) -> (w912:T3)
            n408 = Enqueue Element(queue=w905, element=w903, error in (no error)=w904) -> (queue out=w902:refnum<queue>, error out=w901:errorcluster)  [unwired: 1 in, 1 out]
          }
          frame "Arduino_Close" {
            n409 = property on="Arduino" class="Bool (strict)"() -> (error out=w920:errorcluster, "Value"=w919:bool)  [unwired: 2 in, 1 out]
            n410 = Unbundle By Name(w923) -> ("Port Arduino"=w927:refnum<visa-resource-name>)
            n411 = property on="Arduino" class="Bool (strict)"(error in=w920, "Value"=FALSE ("Arduino")) -> ()  [unwired: 1 in, 2 out]
            n412 = case shown="False" w919 {
              tunnel: w927 -> [_ w931]
              tunnel: w926 -> [w928 w930]
              tunnel: [w928 w929] -> w925
              frame False {
              }
              frame True {
                n413 = VISA Close(VISA resource name=w931, error in (no error)=w930) -> (error out=w929:errorcluster)
              }
            }
          }
          frame "Arduino_LoadProgram" {
            n414 = Unbundle By Name(w936) -> ("Spin Program"=w935:dbl[][], "Numeric 1"=w933:dbl)
            n415 = Unbundle By Name(w938) -> ("Port Arduino"=w940:refnum<visa-resource-name>)
            n416 = node(w933) -> (w932:dbl[unit])
            n417 = call "SpinCoaterArray2String_v02.vi"("Time Start"=w932, "Program Spin Coater\nSpeed (rpm)          Time (s)"=w935) -> ("remote control String"=w934:string)  [unwired: 3 in]
            n418 = VISA Write(VISA resource name=w940, write buffer=w934, error in (no error)=w941) -> (error out=w937:errorcluster)  [unwired: 2 out]
          }
          frame "Arduino_StartProgram" {
            n419 = Unbundle By Name(w949) -> ("Port Arduino"=w948:refnum<visa-resource-name>)
            n420 = VISA Write(VISA resource name=w948, write buffer="run", error in (no error)=w946) -> (error out=w945:errorcluster)  [unwired: 2 out]
            n421 = property on="Action" class="Str"("Value"="Measuring" ("Action")) -> ()  [unwired: 2 in, 2 out]
          }
          frame "Arduino_SetSpeed" {
            n422 = Unbundle By Name(w959) -> ("Numeric 1"=w957:dbl)
            n423 = Unbundle By Name(w961) -> ("Port Arduino"=w960:refnum<visa-resource-name>)
            n424 = To Unsigned Long Integer(number=w957) -> (unsigned 32bit integer=w956:u32)
            n425 = Number To Decimal String(number=w956) -> (decimal integer string=w955:string)  [unwired: 1 in]
            n426 = Concatenate Strings("!spe" ("string"), w955) -> (w953:string)
            n427 = VISA Write(VISA resource name=w960, write buffer=w953, error in (no error)=w958) -> (error out=w952:errorcluster)  [unwired: 2 out]
          }
          frame "Arduino_SetMillis" {
            n428 = Unbundle By Name(w965) -> ("Numeric 1"=w973:dbl)
            n429 = Unbundle By Name(w963) -> ("Port Arduino"=w974:refnum<visa-resource-name>)
            n430 = To Unsigned Long Integer(number=w973) -> (unsigned 32bit integer=w972:u32)
            n431 = Number To Decimal String(number=w972) -> (decimal integer string=w971:string)  [unwired: 1 in]
            n432 = Concatenate Strings("!mil" ("string"), w971) -> (w969:string)
            n433 = VISA Write(VISA resource name=w974, write buffer=w969, error in (no error)=w968) -> (error out=w966:errorcluster)  [unwired: 2 out]
          }
          frame "Arduino_StopSpin" {
            n434 = Unbundle By Name(w978) -> ("Port Arduino"=w977:refnum<visa-resource-name>)
            n435 = VISA Write(VISA resource name=w977, write buffer="abo", error in (no error)=w979) -> (error out=w975:errorcluster)  [unwired: 2 out]
          }
          frame "Measure_Stop" {
            w988 = T4 {"QueueAction"=enum."TimeOut", "Data"=[], "Data_Raw"=[], "Data_Dark"=[], "Data_Ref"=[], "Device Information"=[], "Numeric Control"=0.0, "Boolean"=FALSE, "Wavelength"=[], "Time"=[], "Time Stamp"=timestamp(0 s since 1904-01-01), "Numeric Control 2"=0.0}  # DataQueue
            n436 = Bundle By Name(cluster=w988, "QueueAction"=DataQueue_Action."Stop_Measurement") -> (w989:T4)
            n437 = Enqueue Element(queue=w986, element=w989, error in (no error)=w983) -> (queue out=w985:refnum<queue>, error out=w982:errorcluster)  [unwired: 1 in, 1 out]
          }
          frame "Measure_InSitu" {
            w1030 = T6 {"QueueAction"=enum."TimeOut", "Numeric 1"=0.0, "Numeric 2"=0.0, "Boolean 1"=FALSE, "Boolean 2"=FALSE, "Spin Program"=[]}  # Device Queue
            w1037 = T6 {"QueueAction"=enum."TimeOut", "Numeric 1"=0.0, "Numeric 2"=0.0, "Boolean 1"=FALSE, "Boolean 2"=FALSE, "Spin Program"=[]}  # Device Queue
            n438 = Bundle By Name(cluster=w1037, "QueueAction"=DeviceQueue_Action."Spectrometer_SetTriggerMode", "Numeric 1"=1.0) -> (w1035:T6)
            n439 = Bundle By Name(cluster=w1030, "QueueAction"=DeviceQueue_Action."Spectrometer_DeviceInformation") -> (w1027:T6)
            n440 = Bundle By Name(cluster=w1027, "QueueAction"=DeviceQueue_Action."Spectrometer_StartMeasurement") -> (w1023:T6)
            n441 = Enqueue Element(queue=w1036, element=w1035, error in (no error)=w992) -> (queue out=w1032:refnum<queue>, error out=w1033:errorcluster)  [unwired: 1 in, 1 out]
            n442 = property on="Frames" class="DigNum (strict)"() -> ("Value"=w993:i32)  [unwired: 2 in, 2 out]
            n443 = Bundle By Name(cluster=w1023, "QueueAction"=DeviceQueue_Action."Arduino_StartProgram") -> (w1018:T6)
            n444 = Enqueue Element(queue=w1032, element=w1027, error in (no error)=w1033) -> (queue out=w1029:refnum<queue>, error out=w1028:errorcluster)  [unwired: 1 in, 1 out]
            n445 = Bundle By Name(cluster=w1018, "QueueAction"=DeviceQueue_Action."Spectrometer_GetData", "Numeric 1"="Dividider Get Spectra") -> (w1013:T6)
            n446 = Divide(x=w993, y="Dividider Get Spectra") -> (x/y=w1025:dbl)
            n447 = Round Toward +Infinity(x=w1025) -> (ceil(x): smallest int >= x=w1024:dbl)
            n448 = Enqueue Element(queue=w1029, element=w1023, error in (no error)=w1028) -> (queue out=w1022:refnum<queue>, error out=w1021:errorcluster)  [unwired: 1 in, 1 out]
            n449 = Enqueue Element(queue=w1022, element=w1018, error in (no error)=w1021) -> (queue out=w1019:refnum<queue>, error out=w1016:errorcluster)  [unwired: 1 in, 1 out]
            n450 = for {
              N: w1024 -> [_]
              shift-right: [w1040] -> w1015
              shift-left: w1019 -> [w1044]
              tunnel: w1013 -> [w1041]
              shift-right: [w1042] -> w1014
              shift-left: w1016 -> [w1043]
              n451 = Enqueue Element(queue=w1044, element=w1041, error in (no error)=w1043) -> (queue out=w1040:refnum<queue>, error out=w1042:errorcluster)  [unwired: 1 in, 1 out]
            }
            n452 = Bundle By Name(cluster=w1013, "QueueAction"=DeviceQueue_Action."Spectrometer_StopMeasurement") -> (w1009:T6)
            n453 = property on="Frames for Spectrometer" class="DigNum (strict)"() -> ("Value"=w995:dbl)  [unwired: 2 in, 2 out]
            n454 = Bundle By Name(cluster=w1009, "QueueAction"=DeviceQueue_Action."Measure_Stop") -> (w1002:T6)
            n455 = Enqueue Element(queue=w1015, element=w1009, error in (no error)=w1014) -> (queue out=w1010:refnum<queue>, error out=w1011:errorcluster)  [unwired: 1 in, 1 out]
            n456 = Bundle By Name(cluster=w1002, "QueueAction"=DeviceQueue_Action."Spectrometer_SetTriggerMode", "Numeric 1"=0.0) -> (w997:T6)
            n457 = Enqueue Element(queue=w1010, element=w1002, error in (no error)=w1011) -> (queue out=w1005:refnum<queue>, error out=w1006:errorcluster)  [unwired: 1 in, 1 out]
            n458 = Bundle By Name(cluster=w997, "QueueAction"=DeviceQueue_Action."Spectrometer_SetFrames", "Numeric 1"=w995) -> (w994:T6)
            n459 = Enqueue Element(queue=w1005, element=w997, error in (no error)=w1006) -> (queue out=w1004:refnum<queue>, error out=w1003:errorcluster)  [unwired: 1 in, 1 out]
            n460 = Enqueue Element(queue=w1004, element=w994, error in (no error)=w1003) -> (queue out=w998:refnum<queue>, error out=w999:errorcluster)  [unwired: 1 in, 1 out]
          }
          frame "Measure_Spectrum" {
            w1057 = T6 {"QueueAction"=enum."TimeOut", "Numeric 1"=0.0, "Numeric 2"=0.0, "Boolean 1"=FALSE, "Boolean 2"=FALSE, "Spin Program"=[]}  # Device Queue
            n461 = Bundle By Name(cluster=w1057, "QueueAction"=DeviceQueue_Action."Spectrometer_Measure") -> (w1049:T6)
            n462 = Bundle By Name(cluster=w1049, "QueueAction"=DeviceQueue_Action."Measure_Stop") -> (w1047:T6)
            n463 = Enqueue Element(queue=w1055, element=w1049, error in (no error)=w1054) -> (queue out=w1050:refnum<queue>, error out=w1051:errorcluster)  [unwired: 1 in, 1 out]
            n464 = Enqueue Element(queue=w1050, element=w1047, error in (no error)=w1051) -> (queue out=w1046:refnum<queue>, error out=w1045:errorcluster)  [unwired: 1 in, 1 out]
          }
        }
      }
      frame Error {
        w1062 = T14 4 items=["no dialog", "OK message", "continue or stop message", "OK message + warnings", "continue/stop + warnings"] ("type of dialog (OK msg:1)")
        n465 = call <vilib>:"General Error Handler.vi"("type of dialog (OK msg:1)"=w1062, "error in (no error)"=w1063) -> ("error out"=w1061:errorcluster)  [unwired: 9 in, 4 out]
        n466 = call <vilib>:"Clear Errors.vi"("error in (no error)"=w1061) -> ("error out"=w1060:errorcluster)  [unwired: 5 in, 1 out]
      }
    }
  }
  n467 = disable-structure shown="Enabled" {
    frame Disabled {
      w1066 = T6 {"QueueAction"=enum."TimeOut", "Numeric 1"=0.0, "Numeric 2"=0.0, "Boolean 1"=FALSE, "Boolean 2"=FALSE, "Spin Program"=[]}  # Device Queue
      n468 = Bundle By Name(cluster=w1066, "QueueAction"=DeviceQueue_Action."Arduino_SetSpeed") -> (w1065:T6)  [unwired: 1 in]
      n469 = Enqueue Element(element=w1065) -> ()  [unwired: 3 in, 3 out]
    }
    frame Enabled {
    }
  }
  n470 = Release Queue(queue=w9) -> ()  [unwired: 2 in, 3 out]
  n471 = Release Queue(queue=w10) -> ()  [unwired: 2 in, 3 out]
